vi "CIPT_softwarecontrol auto probe 9 8 23.vi"() -> ()   [LabVIEW 2022 SP3]
uses:
  Git/CIPT/CIPT/Labview Project/CIPT modes.ctl
  <vilib>/Analysis/baseanly.llb/Mean (DBL).vi
  <vilib>/Utility/file.llb/Read Delimited Spreadsheet (DBL).vi
  <vilib>/Utility/file.llb/Read Delimited Spreadsheet (I64).vi
  <vilib>/gmath/NumericalOptimization/Nonlinear Curve Fit LM.vi
  <vilib>/Utility/file.llb/Write Delimited Spreadsheet (string).vi
  <vilib>/Utility/file.llb/Write Delimited Spreadsheet (I64).vi
  <vilib>/Utility/file.llb/Write Delimited Spreadsheet (DBL).vi
  C:/CIPT/Labview Project/Camera Driver/Labview Driver/OtherDrivers/LabVIEW/ueye.NET/uEyeDotNet.dll
  CIPT/Labview Project/Camera Driver/Labview Driver/OtherDrivers/LabVIEW/ueye.NET/uEyeDotNet.dll
  <vilib>/gmath/NI_Gmath.lvlib
  <instrlib>/Keithley DMM6500 DAQ6500 Series/Keithley DMM6500 DAQ6500 Series.lvlib
  <instrlib>/Keithley 24XX/Keithley 24XX.lvlib
  <instrlib>/Keithley 2182/Keithley 2182.lvlib
  <vilib>/Analysis/NI_AALBase.lvlib
panel:
  out "Comms Errors":errorcluster[](array[cluster])
  in  "Save File":bool
  out "error file out":errorcluster
  in  "output file path":path=path "C:/CIPT/Labview Project/csv files/test output.csv"
  in  "stop":bool
  in  "Tab Control":T1(tab)
  in  "Camera ID 3":enum16{"2", "1"}(ring)
  in  "Camera ID 1":enum16{"2", "1"}(ring)
  in  "down a2":bool
  in  "up a2":bool
  in  "down a1":bool
  in  "up a1":bool
  in  "down a3":bool
  in  "up a3":bool
  in  "down all":bool
  in  "up all":bool
  in  "steps /\n continuous \ntoggle":bool
  out "Image first camera":picture
  out "Serial Number 1":string
  in  "Init Camera":bool
  in  "Exit Camera":bool
  in  "Init Camera 2":bool
  in  "Exit Camera 2":bool
  out "Serial Number 2":string
  out "Image second camera":picture
  out "Error Camera 1":errorcluster caption="error"
  out "Error Camera 2":errorcluster caption="error"
  in  "COM 1 (motor)":refnum<visa-resource-name>="COM1"
  out "error":errorcluster
  in  "Turn On Landing Test":bool
  in  "Step size":i32=10
  in  "Probe Landing File":path=path "C:/CIPT/Labview Project/csv files/Probe Landing cipt.csv"
  out "List Of Probe Configs":i64[][](array[numeric])
  out "Resistance For Each Relay Config":sgl[](array[numeric])
  in  "Probe Threshold (ohm)":dbl=100000.0
  out "Touching Probes Configs":i64[][](array[numeric])
  in  "Automatically Move Probe to Surface":bool
  out "Loaded":bool
  out "Loaded":bool
  out "Error Probe Configuration File":errorcluster
  in  "Probe Configuration File":path=path "C:/CIPT/Labview Project/csv files/test probe config.csv"
  in  "Probe Settings File":path=path "C:/CIPT/Labview Project/csv files/deafult_probe_setrings.CSV"
  out "Error Probe Settings File":errorcluster
  out "Probe Spacings":dbl[][](array[numeric])
  in  "Load":bool
  in  "Multiplexer":refnum<visa-resource-name>
  out "all rows":i64[][](array[numeric])
  out "Results Description":string[](array[string])
  out "Results":dbl[][](array[numeric])
  out "Probe Set 2":i32
  in  "Compliance voltage (V)":dbl=42.0
  in  "Measure Instrument":refnum<visa-resource-name>
  in  "Radio Buttons":T2 caption="Select Instrumentation"
  in  "Source Instrument":refnum<visa-resource-name>="Sourcemeter"
  in  "Run":bool
  in  "Current (µA)":dbl=10.0
  out "Measurement Log":string
  out "Probe Set":i32
  in  "Measurement Repeats":i32=10
  in  "Size Of Buffer Used For One Measurement":i32=3
  in  "Top Film R est.":dbl=0.25
  in  "Bottm Film R est.":dbl=0.25
  in  "RA est.":dbl=0.25
  out "Top Film R":dbl
  out "Bottom Film R":dbl
  out "RA":dbl
  out "error out (fitting model)":errorcluster
  in  "Fit Data":bool
  out "Measurements Map Out":map{string, dbl[]}(c390)
  # "Probe Landing cipt_probe check: checks probes individually \nProbe Landing cipt: checks for any connection"
  # "All"
  # "End"
  # "Home"
  # "Delete"
  # "Insert"
  # "Page Down"
  # "Page Up"
  # "F2"
  # "F1"
  # "Steps"
  # "Continuous"
  # "Probe Settings"
  # "Probe Configuration"
  # "I+"
  # "V+"
  # "V-"
  # "I-"
  # "Max Resolution of 2400 is 300 µV in 200 mV range"
  # "/"
  # "Sheet Resistance (RA)"
  # "Estimated Values"
  # "Fitted Values"
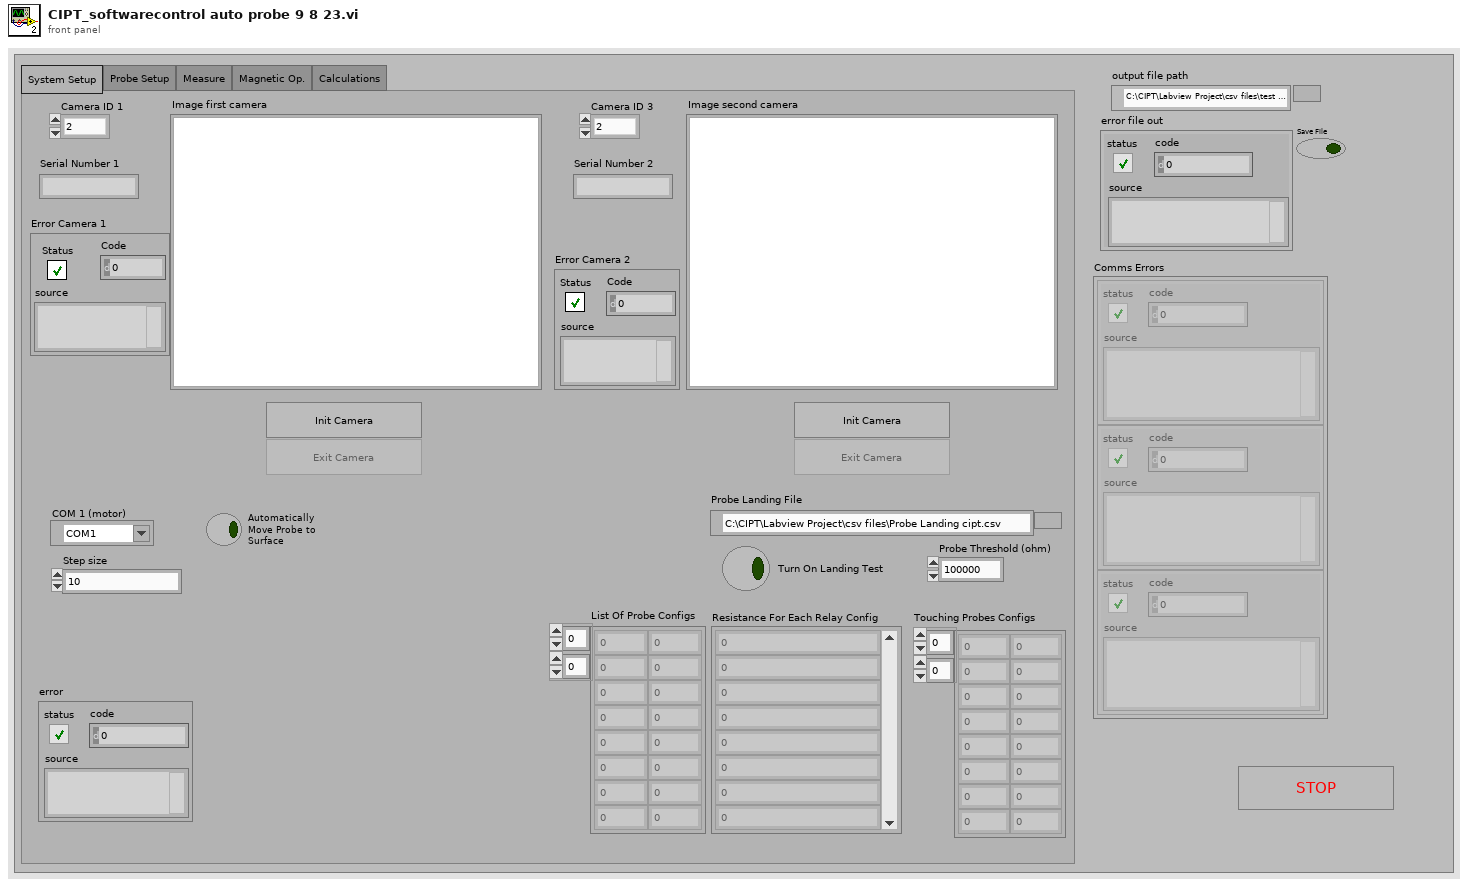
[diagram p1: front panel]
types:
  T1 = enum32{"System Setup", "Probe Setup", "Measure", "Magnetic Op.", "Calculations"}
  T2 = typedef "CIPT modes.ctl" = enum32{"DAQ6510", "2400 Only", "2400 and  2182", "SR830", "SR830 and 6221"}
  T3 = enum32{"System Setup", "Probe Setup", "Measure", "Magnetic Operations", "Calculations + Analyis"}
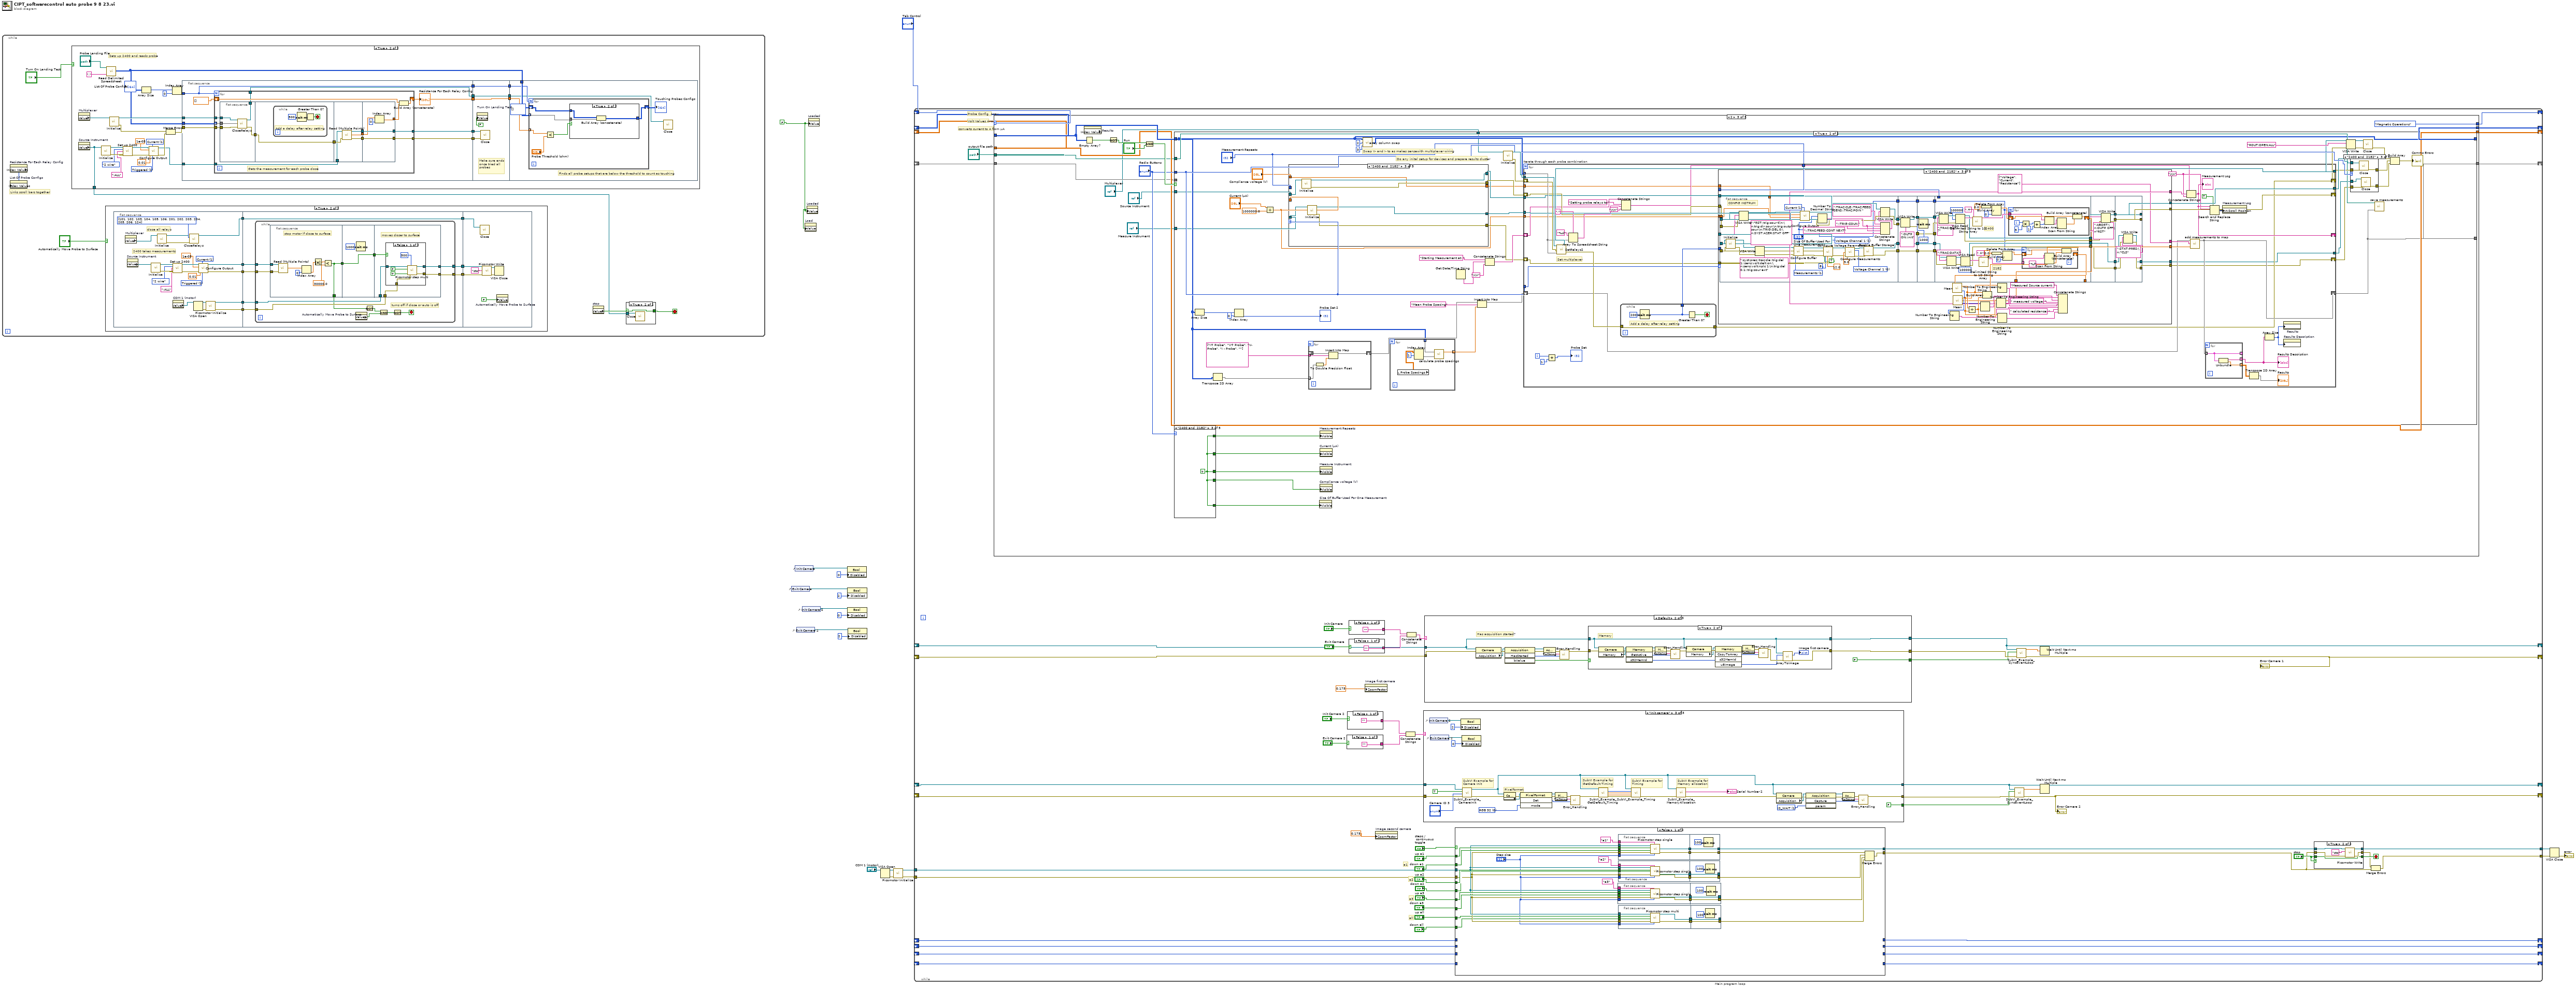
[diagram p0: block diagram]
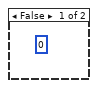
[diagram p5: hidden frame]
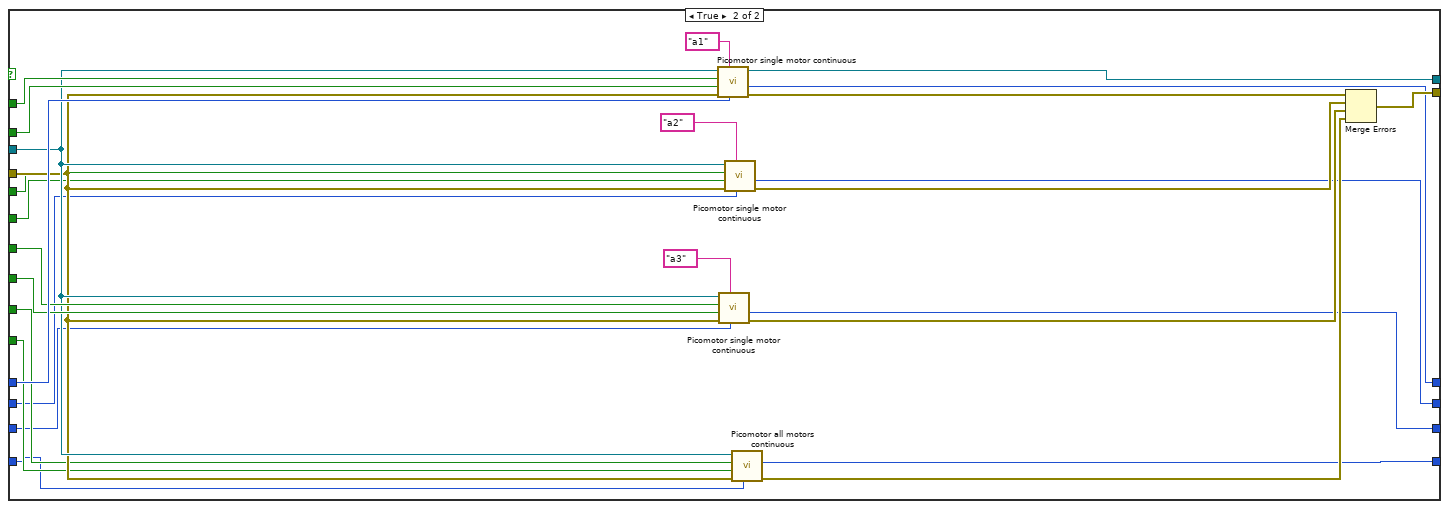
[diagram p7: hidden frame]
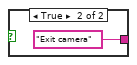
[diagram p9: hidden frame]
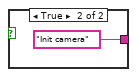
[diagram p10: hidden frame]
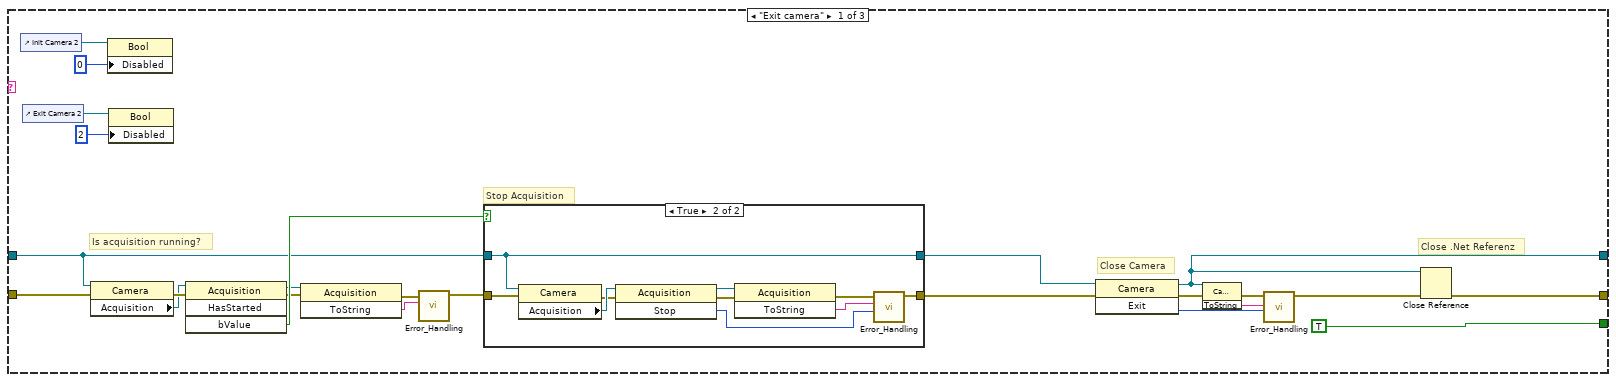
[diagram p11: hidden frame]
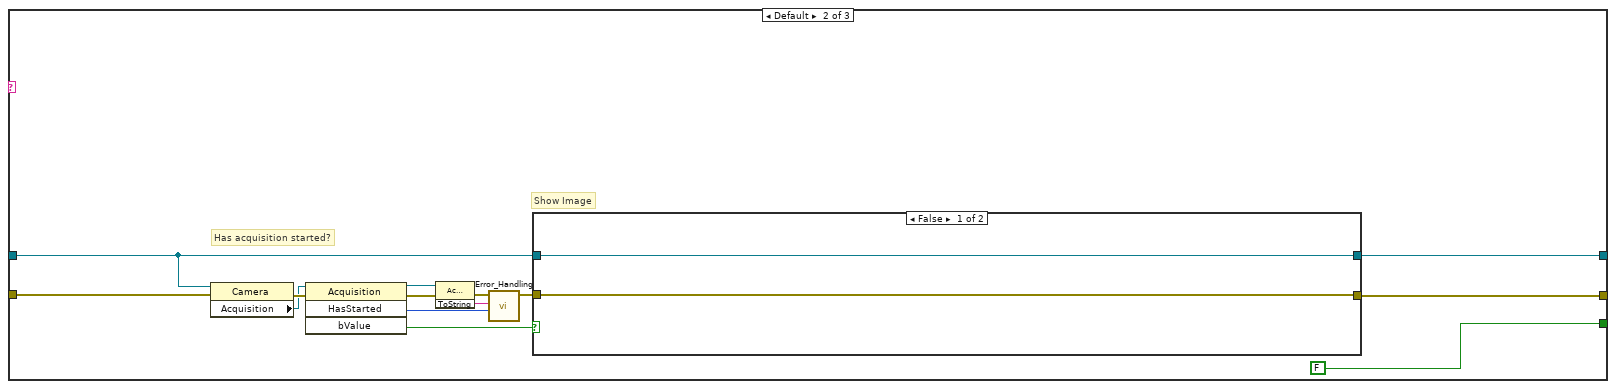
[diagram p13: hidden frame]
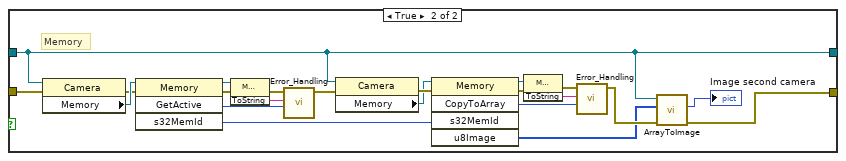
[diagram p14: hidden frame]
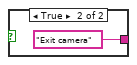
[diagram p15: hidden frame]
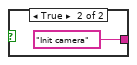
[diagram p16: hidden frame]
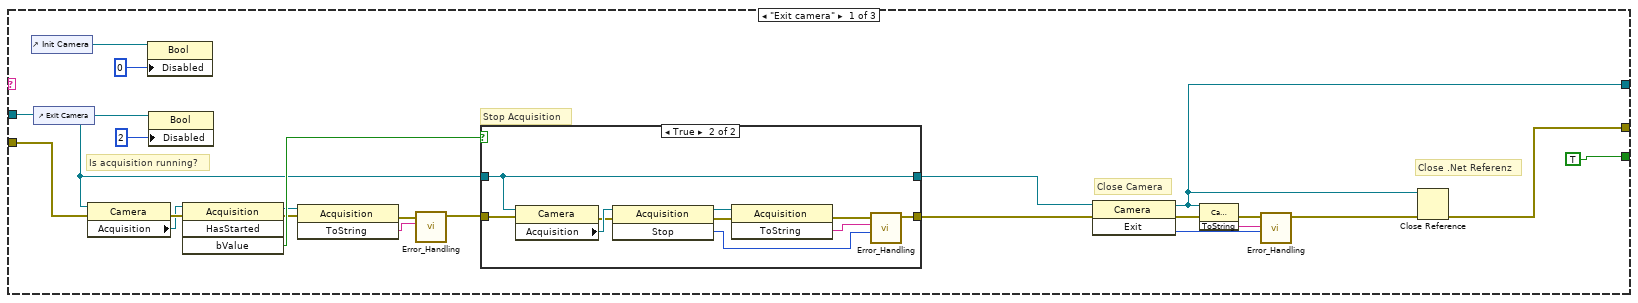
[diagram p17: hidden frame]
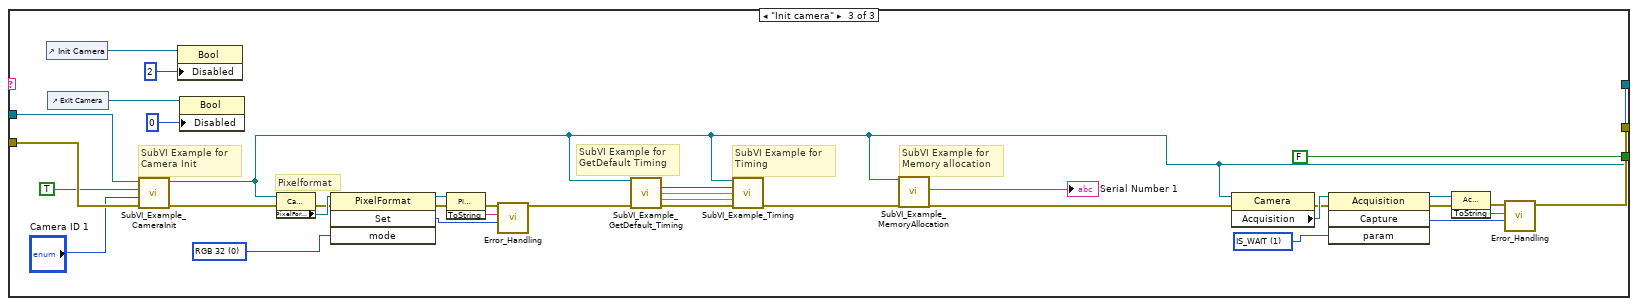
[diagram p20: hidden frame]
diagram:
  w9 = FALSE
  n1 = while {
    stop <- w24 stop-if-true
    # "Links scroll bars together"
    n2 = property on="Resistance For Each Relay Config" class="Arr (strict)"() -> ("Index Values"=w20:u32[])  [unwired: 2 in, 2 out]
    n3 = property on="List Of Probe Configs" class="Arr (strict)"("Index Values"=w20) -> ()  [unwired: 2 in, 2 out]
    n4 = case shown="True" "Turn On Landing Test" {
      tunnel: [_ w117] -> w21
      frame False {
        (unwired) 0
      }
      frame True {
        w134 = u16 1 items=["Immediate", "Triggered"] ("Output Type  (0: Immediate)")
        w133 = u16 1 items=["Voltage", "Current"] ("Source Mode  (0: Voltage)")
        # "Sets up 2400 and reads probe"
        n5 = property on="Multiplexer" class="VISAName"() -> ("Value"=w128:refnum<visa-resource-name>)  [unwired: 2 in, 2 out]
        n6 = property on="Source Instrument" class="VISAName"() -> ("Value"=w117:refnum<visa-resource-name>)  [unwired: 2 in, 2 out]
        n7 = call <instrlib>:"Initialize.vi"("VISA resource name"=w117) -> ("error out"=w136:errorcluster, "VISA resource name out"=w135:refnum<visa-resource-name>)  [unwired: 9 in]
        n8 = call-poly <vilib>:"Read Delimited Spreadsheet.vi"("file path (dialog if empty)"="Probe Landing File", "delimiter (\\t)"="," ("delimiter (\\t)")) -> ("all rows"=w114:i64[][])  [unwired: 8 in, 5 out]
        "List Of Probe Configs" <- w114
        n9 = call <instrlib>:"Initialize.vi"("VISA resource name"=w128) -> ("error out"=w126:errorcluster, "VISA resource name out"=w121:refnum<visa-resource-name>)  [unwired: 9 in]
        n10 = call "Set up 2400.vi"("VISA resource name"=w135, "Sense mode"=enum16{"2 wire", "4 wire"}."2 wire", "Measurement Function"=":ALL", "error in (no error)"=w136) -> ("VISA resource name out"=w137:refnum<visa-resource-name>, "error out"=w138:errorcluster)  [unwired: 10 in]
        n11 = Array Size(array=w114) -> (size(s)=w125:i32[])
        n12 = call <instrlib>:"Configure Output.vi"("Output Type  (0: Immediate)"=w134, "Source Mode  (0: Voltage)"=w133, "error in (no error)"=w138, "Compliance  Level (0.1)"=0.01, "Output Level (0)"=1e-05, "VISA resource name"=w137) -> ("error out"=w127:errorcluster, "VISA resource name out"=w120:refnum<visa-resource-name>)  [unwired: 4 in]
        n13 = Merge Errors(w126, w127) -> (w122:errorcluster)
        n14 = Index Array(array=w125, index=0) -> (element=w123:i32)
        n15 = flat-sequence {
          tunnel: w123 -> [w143]
          tunnel: w122 -> [w150]
          tunnel: w121 -> [w149]
          tunnel: w114 -> [w148]
          tunnel: w120 -> [w147]
          tunnel: [w146] -> w119
          tunnel: [w145] -> w118
          tunnel: [w144] -> w115
          tunnel: [w143] -> w112
          tunnel: [w141] -> w110
          tunnel: w119 -> [w189]
          tunnel: w118 -> [w188]
          tunnel: [w187] -> w116
          tunnel: w115 -> [w187]
          tunnel: [w186] -> w113
          tunnel: w112 -> [w186]
          tunnel: [w185] -> w111
          tunnel: w110 -> [w185]
          tunnel: w116 -> [w196]
          tunnel: w114 -> [w195]
          tunnel: w113 -> [w194]
          tunnel: w111 -> [w191]
          frame #0 {
            n16 = for {
              N: w143 -> [_]
              tunnel: w150 -> [w163]
              tunnel: w149 -> [w162]
              tunnel: w148 -> [w161] mode=indexing
              shift-right: [w156] -> w144
              shift-left: dbl[] [] -> [w155]
              tunnel: w147 -> [w154]
              tunnel: [w153] -> w146
              tunnel: [w152] -> w145
              tunnel: [w151] -> w141
              # "Gets the measurement for each probe close"
              n17 = flat-sequence {
                tunnel: [w170] -> w165
                tunnel: w163 -> [w169]
                tunnel: w162 -> [w168]
                tunnel: w161 -> [w167]
                tunnel: [w166] -> w151
                tunnel: [w171] -> w164
                tunnel: w165 -> [w171]
                tunnel: w164 -> [w179]
                tunnel: [w178] -> w160
                tunnel: [w177] -> w159
                tunnel: [w176] -> w158
                tunnel: w154 -> [w175]
                tunnel: [w183] -> w152
                tunnel: [w184] -> w153
                tunnel: w160 -> [w184]
                tunnel: w159 -> [w183]
                tunnel: w158 -> [w181]
                tunnel: [w180] -> w157
                frame #0 {
                  n18 = call "CloseRelays.vi"("error in (no error)"=w169, "Array"=w167, "VISA Refnum in"=w168) -> ("error out"=w170:errorcluster, "VISA Refnum out"=w166:refnum<visa-resource-name>)  [unwired: 6 in, 1 out]
                }
                frame #1 {
                  n19 = while {
                    stop <- w173 stop-if-true
                    # "Add a delay after relay setting"
                    n20 = Wait (ms)(milliseconds to wait=u32 500) -> (millisecond timer value=w172:u32)
                    n21 = Greater Than 0?(x=w172) -> (x > 0?=w173:bool)
                  }
                }
                frame #2 {
                  n22 = call <instrlib>:"Read (Multiple Points).vi"("VISA resource name"=w175, "error in (no error)"=w179) -> ("VISA resource name out"=w178:refnum<visa-resource-name>, "Resistance"=w176:sgl[], "error out"=w177:errorcluster)  [unwired: 7 in, 4 out]
                }
                frame #3 {
                  n23 = Index Array(array=w181, index=0) -> (element=w180:sgl)
                }
              }
              n24 = Build Array (concatenate)(w155, w157) -> (w156:dbl[])
            }
            "Resistance For Each Relay Config" <- w144
          }
          frame #1 {
            # "Make sure ends once tried all probes"
            n25 = property on="Turn On Landing Test" class="Bool (strict)"("Value"=FALSE) -> ()  [unwired: 2 in, 2 out]
            n26 = call <instrlib>:"Close.vi"("error in (no error)"=w188, "VISA resource name"=w189) -> ()  [unwired: 9 in, 1 out]
          }
          frame #2 {
            # "Finds all probe setups that are below the threshold to count as touching"
            n27 = for {
              N: w194 -> [_]
              tunnel: w196 -> [w201] mode=indexing
              tunnel: w195 -> [w199] mode=indexing
              shift-right: [w198] -> w193
              shift-left: i64[][] [] -> [w197]
              n28 = Less?(x=w201, y="Probe Threshold (ohm)") -> (x < y?=w200:bool)
              n29 = case shown="True" w200 {
                tunnel: w199 -> [_ w206]
                tunnel: [w203 w205] -> w198
                tunnel: w197 -> [w203 w204]
                frame False {
                }
                frame True {
                  n30 = Build Array (concatenate)(w204, w206) -> (w205:i64[][])
                }
              }
            }
            "Touching Probes Configs" <- w193
            n31 = call <instrlib>:"Close.vi"("VISA resource name"=w191) -> ()  [unwired: 10 in, 1 out]
          }
        }
      }
    }
    n32 = case shown="True" "Automatically Move Probe to Surface" {
      frame False {
      }
      frame True {
        n33 = flat-sequence {
          tunnel: [w42] -> w32
          tunnel: [w41] -> w31
          tunnel: [w37] -> w30
          tunnel: [w36] -> w29
          tunnel: [w35] -> w28
          tunnel: w32 -> [w61]
          tunnel: w31 -> [w60]
          tunnel: w30 -> [w59]
          tunnel: w29 -> [w58]
          tunnel: w28 -> [w62]
          tunnel: [w62] -> w27
          tunnel: [w57] -> w26
          tunnel: [w56] -> w25
          tunnel: w27 -> [w101]
          tunnel: w26 -> [w102]
          tunnel: w25 -> [w104]
          frame #0 {
            w51 = u16 1 items=["Immediate", "Triggered"] ("Output Type  (0: Immediate)")
            w33 = u16 1 items=["Voltage", "Current"] ("Source Mode  (0: Voltage)")
            # "2400 takes measurements"
            # "close all relays"
            n34 = property on="Multiplexer" class="VISAName"() -> ("Value"=w46:refnum<visa-resource-name>)  [unwired: 2 in, 2 out]
            n35 = property on="Source Instrument" class="VISAName"() -> ("Value"=w47:refnum<visa-resource-name>)  [unwired: 2 in, 2 out]
            n36 = call <instrlib>:"Initialize.vi"("VISA resource name"=w47) -> ("error out"=w53:errorcluster, "VISA resource name out"=w52:refnum<visa-resource-name>)  [unwired: 9 in]
            n37 = call <instrlib>:"Initialize.vi"("VISA resource name"=w46) -> ("error out"=w43:errorcluster, "VISA resource name out"=w44:refnum<visa-resource-name>)  [unwired: 9 in]
            n38 = call "Set up 2400.vi"("VISA resource name"=w52, "Sense mode"=enum16{"2 wire", "4 wire"}."2 wire", "Measurement Function"=":ALL", "error in (no error)"=w53) -> ("VISA resource name out"=w54:refnum<visa-resource-name>, "error out"=w55:errorcluster)  [unwired: 10 in]
            n39 = property on="COM 1 (motor)" class="VISAName"() -> ("Value"=w40:refnum<visa-resource-name>)  [unwired: 2 in, 2 out]
            n40 = call "CloseRelays.vi"("error in (no error)"=w43, "Array"=i32[] [101, 102, 103, 104, 105, 106, 201, 202, 203, 204, 205, 206, 124], "VISA Refnum in"=w44) -> ("VISA Refnum out"=w35:refnum<visa-resource-name>)  [unwired: 6 in, 2 out]
            n41 = VISA Open(VISA resource name=w40) -> (VISA resource name=w38:refnum<visa-resource-name>, error out=w39:errorcluster)  [unwired: 4 in]
            n42 = call <instrlib>:"Configure Output.vi"("Output Type  (0: Immediate)"=w51, "Source Mode  (0: Voltage)"=w33, "error in (no error)"=w55, "Compliance  Level (0.1)"=0.01, "Output Level (0)"=1e-05, "VISA resource name"=w54) -> ("error out"=w41:errorcluster, "VISA resource name out"=w42:refnum<visa-resource-name>)  [unwired: 4 in]
            n43 = call "Picomotor Initialize.vi"("error in (no error)"=w39, "VISA Refnum in"=w38) -> ("error out"=w36:errorcluster, "VISA Refnum out"=w37:refnum<visa-resource-name>)  [unwired: 8 in]
          }
          frame #1 {
            n44 = while {
              tunnel: w61 -> [w75]
              tunnel: w60 -> [w74]
              tunnel: w59 -> [w73]
              tunnel: w58 -> [w72]
              tunnel: [w71] -> w57
              tunnel: [w70] -> w56
              stop <- w63 stop-if-true
              # "turns off if close or auto is off"
              n45 = flat-sequence {
                tunnel: w75 -> [w81]
                tunnel: w74 -> [w80]
                tunnel: [w78] -> w67
                tunnel: [w78] -> w68
                tunnel: [w84] -> w69
                tunnel: w68 -> [w84]
                tunnel: w73 -> [w89]
                tunnel: w72 -> [w90]
                tunnel: [w87] -> w71
                tunnel: [w88] -> w70
                tunnel: w69 -> [w86]
                frame #0 {
                  # "stop motor if close to surface"
                  n46 = call <instrlib>:"Read (Multiple Points).vi"("VISA resource name"=w81, "error in (no error)"=w80) -> ("Resistance"=w82:sgl[])  [unwired: 7 in, 6 out]
                  n47 = Index Array(array=w82, index=0) -> (element=w77:sgl)
                  n48 = Absolute Value(x=w77) -> (abs(x)=w76:sgl)
                  n49 = Less?(x=w76, y=sgl 30000.0 ("x")) -> (x < y?=w78:bool)
                }
                frame #1 {
                  n50 = Wait (ms)(milliseconds to wait=u32 1000) -> ()  [unwired: 1 out]
                }
                frame #2 {
                  # "moves closer to surface"
                  n51 = case shown="False" w86 {
                    tunnel: w90 -> [w96 w98]
                    tunnel: w89 -> [w93 w99]
                    tunnel: [w92 w98] -> w88
                    tunnel: [w91 w99] -> w87
                    frame False {
                      n52 = call "Picomotor step multi.vi"("Step size"=500, "error in (no error)"=w96, "down a1"=TRUE, "up a1"=FALSE, "VISA Refnum in"=w93) -> ("error out"=w92:errorcluster, "VISA Refnum out"=w91:refnum<visa-resource-name>)  [unwired: 5 in]
                    }
                    frame True {
                    }
                  }
                }
              }
              n53 = property on="Automatically Move Probe to Surface" class="Bool (strict)"() -> ("Value"=w66:bool)  [unwired: 2 in, 2 out]
              n54 = Not(x=w67) -> (.not. x?=w65:bool)
              n55 = And(x=w65, y=w66) -> (x .and. y?=w64:bool)
              n56 = Not(x=w64) -> (.not. x?=w63:bool)
            }
          }
          frame #2 {
            n57 = call <instrlib>:"Close.vi"("VISA resource name"=w101) -> ()  [unwired: 10 in, 1 out]
            n58 = call "Picomotor Write.vi"("error in (no error)"=w104, "String 3"="sto", "VISA Refnum in"=w102) -> ("error out"=w106:errorcluster, "VISA Refnum out"=w105:refnum<visa-resource-name>)  [unwired: 6 in, 1 out]
            n59 = VISA Close(VISA resource name=w105, error in (no error)=w106) -> ()  [unwired: 1 out]
            n60 = property on="Automatically Move Probe to Surface" class="Bool (strict)"("Value"=FALSE) -> ()  [unwired: 2 in, 2 out]
          }
        }
      }
    }
    n61 = property on="stop" class="Bool (strict)"() -> ("Value"=w22:bool)  [unwired: 2 in, 2 out]
    n62 = case shown="True" w22 {
      selector: w22 -> [w107 w109]
      tunnel: [w107 w109] -> w24
      tunnel: w21 -> [_ w108]
      frame False {
      }
      frame True {
        n63 = call <instrlib>:"Close.vi"("VISA resource name"=w108) -> ()  [unwired: 10 in, 1 out]
      }
    }
  }
  n64 = control-ref of="Exit Camera"() -> (w12:refnum<vi>)
  n65 = control-ref of="Init Camera"() -> (w13:refnum<vi>)
  n66 = control-ref of="Exit Camera 2"() -> (w17:refnum<vi>)
  n67 = control-ref of="Init Camera 2"() -> (w16:refnum<vi>)
  n68 = property on="Load" class="Bool (strict)"("Value"=w9) -> ()  [unwired: 2 in, 2 out]
  n69 = property on="Loaded" class="Bool (strict)"("Value"=w9) -> ()  [unwired: 2 in, 2 out]
  n70 = property on="Loaded" class="Bool (strict)"("Value"=w9) -> ()  [unwired: 2 in, 2 out]
  n71 = property class="Bool"(reference=w13, "Disabled"=u8 0 ("Deaktiviert")) -> ()  [unwired: 1 in, 2 out]
  n72 = property class="Bool"(reference=w12, "Disabled"=u8 2 ("Deaktiviert")) -> ()  [unwired: 1 in, 2 out]
  n73 = property class="Bool"(reference=w16, "Disabled"=u8 0 ("Deaktiviert")) -> ()  [unwired: 1 in, 2 out]
  n74 = property class="Bool"(reference=w17, "Disabled"=u8 2 ("Deaktiviert")) -> ()  [unwired: 1 in, 2 out]
  n75 = VISA Open(VISA resource name="COM 1 (motor)") -> (VISA resource name=w7:refnum<visa-resource-name>, error out=w6:errorcluster)  [unwired: 4 in]
  n76 = call "Picomotor Initialize.vi"("error in (no error)"=w6, "VISA Refnum in"=w7) -> ("error out"=w4:errorcluster, "VISA Refnum out"=w5:refnum<visa-resource-name>)  [unwired: 8 in]
  n77 = while "Main program loop" {
    shift-right: [w265] -> _
    shift-left: _ -> [w266]
    shift-right: [w264] -> _
    shift-left: "Tab Control" -> [w267]
    shift-right: [w263] -> _
    shift-left: _ -> [w262]
    shift-right: [w260] -> _
    shift-left: _ -> [w259]
    shift-right: [w248] -> _
    shift-left: _ -> [w246]
    shift-right: [w249] -> _
    shift-left: _ -> [w247]
    shift-right: [w236] -> _
    shift-left: _ -> [w234]
    shift-right: [w235] -> _
    shift-left: _ -> [w233]
    tunnel: w5 -> [w220]
    tunnel: w4 -> [w219]
    tunnel: [w232] -> w2
    shift-right: [w217] -> _
    shift-left: _ -> [w213]
    shift-right: [w216] -> _
    shift-left: _ -> [w212]
    shift-right: [w215] -> _
    shift-left: _ -> [w211]
    shift-right: [w214] -> _
    shift-left: _ -> [w210]
    tunnel: [w207] -> w1
    stop <- w231 stop-if-true
    # "a2"
    # "a3"
    # "all"
    # "a1"
    # "converts current to A from µA"
    # "Volt Values Array"
    # "Probe Config. Array"
    n78 = case shown="2" w267 {
      tunnel: w266 -> [w606 w613 w643 w1002 w1009]
      tunnel: [w606 w617 w642 w1002 w1009] -> w265
      tunnel: [T3."Probe Setup" ("Tab Control") T3."Measure" ("Tab Control") T3."Magnetic Operations" ("Tab Control") T3."Calculations + Analyis" ("Tab Control") T3."System Setup" ("Tab Control")] -> w264
      tunnel: [w604 w612 w637 w1001 w1008] -> w263
      tunnel: w262 -> [w604 w611 w637 w1001 w1008]
      tunnel: "output file path" -> [_ _ w634 _ w1007]
      tunnel: [w603 w608 w633 w1000 w1006] -> w260
      tunnel: w259 -> [w603 w608 w632 w1000 w1006]
      frame 0, Default {
        # "System Setup"
      }
      frame 1 {
        # "Probe Setup"
        n79 = Empty Array?(array=w613) -> (empty?=w607:bool)
        n80 = Empty Array?(array=w611) -> (empty?=w610:bool)
        n81 = Not(x=w607) -> (.not. x?=→"Loaded":bool)
        n82 = Not(x=w610) -> (.not. x?=→"Loaded":bool)
        n83 = case shown="True" "Load" {
          tunnel: [w619 w620] -> w617
          tunnel: w613 -> [w619 _]
          tunnel: [w618 w621] -> w612
          tunnel: w611 -> [w618 _]
          frame False {
          }
          frame True {
            # "Probe config. file and data aquisition"
            # "Probe settings file and data aquisition"
            n84 = call-poly <vilib>:"Read Delimited Spreadsheet.vi"("file path (dialog if empty)"="Probe Configuration File", "delimiter (\\t)"="," ("delimiter (\\t)")) -> ("all rows"=w620:i64[][], "error out"=→"Error Probe Configuration File":errorcluster)  [unwired: 8 in, 4 out]
            "all rows" <- w620
            n85 = call-poly <vilib>:"Read Delimited Spreadsheet.vi"("file path (dialog if empty)"="Probe Settings File", "delimiter (\\t)"="," ("delimiter (\\t)")) -> ("all rows"=w621:dbl[][], "error out"=→"Error Probe Settings File":errorcluster)  [unwired: 8 in, 4 out]
            "Probe Spacings" <- w621
          }
        }
        n86 = property on="Load" class="Bool (strict)"("Value"=w607) -> ()  [unwired: 2 in, 2 out]
      }
      frame 2 {
        n87 = property on="Results" class="Arr (strict)" props=["Index Values"]() -> ()  [unwired: 2 in, 3 out]
        n88 = Empty Array?(array=w643) -> (empty?=w645:bool)
        n89 = Not(x=w645) -> (.not. x?=w644:bool)
        n90 = Compound Arithmetic op=AND(w644, "Run") -> (w647:bool)
        n91 = case shown="True" w647 {
          tunnel: w643 -> [w658 w677]
          tunnel: [w658 w677] -> w642
          tunnel: "Radio Buttons" -> [_ w703]
          tunnel: w634 -> [_ w691]
          tunnel: [w657 w673] -> w633
          tunnel: w632 -> [w657 _]
          tunnel: "Measure Instrument" -> [_ w665]
          tunnel: "Source Instrument" -> [_ w664]
          tunnel: "Multiplexer" -> [_ w663]
          frame False {
          }
          frame True {
            # "Swap V- and I- to as makes sensewith multiplexer wiring"
            # "Do any inital setup for devices and prepare results cluster"
            n92 = Array Size(array=w677) -> (size(s)=w697:i32[])
            n93 = Transpose 2D Array(2D array=w677) -> (transposed array=w676:i64[][])
            n94 = Index Array "Index Array"(array=w697, index=0) -> (element=→"Probe Set 2":i32)
            n95 = Divide(x="Current (µA)", y=1000000.0) -> (x/y=w659:dbl)
            n96 = case shown="\"2400 and  2182\"" w703 {
              tunnel: w664 -> [_ w741 w747 _ _]
              tunnel: [_ w729 w746 _ _] -> w704
              tunnel: w665 -> [_ _ w748 _ _]
              tunnel: [_ w729 w744 _ _] -> w667
              tunnel: [_ w735 w743 _ _] -> w698
              tunnel: w659 -> [_ w732 _ _ _]
              tunnel: "Compliance voltage (V)" -> [_ w730 w742 _ _]
              tunnel: "Measurement Repeats" -> [_ _ _ _ _]
              tunnel: [_ _ w745 _ _] -> w662
              tunnel: [_ _ w742 _ _] -> w660
              frame "DAQ6510", Default {
              }
              frame "2400 Only" {
                w733 = u16 1 items=["Immediate", "Triggered"] ("Output Type  (0: Immediate)")
                w734 = u16 1 items=["Voltage", "Current"] ("Source Mode  (0: Voltage)")
                n97 = call <instrlib>:"Initialize.vi"("VISA resource name"=w741) -> ("error out"=w739:errorcluster, "VISA resource name out"=w740:refnum<visa-resource-name>)  [unwired: 9 in]
                n98 = call "Set up 2400.vi"("VISA resource name"=w740, "Sense mode"=enum16{"2 wire", "4 wire"}."4 wire", "Measurement Function"=":ALL", "error in (no error)"=w739) -> ("VISA resource name out"=w737:refnum<visa-resource-name>, "error out"=w736:errorcluster)  [unwired: 10 in]
                n99 = call <instrlib>:"Configure Output.vi"("Output Type  (0: Immediate)"=w733, "Source Mode  (0: Voltage)"=w734, "error in (no error)"=w736, "Compliance  Level (0.1)"=w730, "Output Level (0)"=w732, "VISA resource name"=w737) -> ("error out"=w735:errorcluster, "VISA resource name out"=w729:refnum<visa-resource-name>)  [unwired: 4 in]
              }
              frame "2400 and  2182" {
                n100 = call <instrlib>:"Initialize.vi"("VISA resource name"=w747) -> ("error out"=w743:errorcluster, "VISA resource name out"=w744:refnum<visa-resource-name>)  [unwired: 9 in]
                n101 = call <instrlib>:"Initialize.vi"("VISA resource name"=w748) -> ("error out"=w745:errorcluster, "VISA resource name out"=w746:refnum<visa-resource-name>)  [unwired: 9 in]
              }
              frame "SR830" {
              }
              frame "SR830 and 6221" {
              }
            }
            n102 = for {
              tunnel: w676 -> [w715] mode=indexing
              tunnel: string[] ["I+ Probe", "V+ Probe", "V- Probe", "I - Probe", ""] -> [w716] mode=indexing
              shift-right: [w713] -> w681
              shift-left: _ -> [w712]
              n103 = To Double Precision Float(number=w715) -> (double precision float=w714:dbl[])
              n104 = Insert Into Map(map in=w712, key=w716, value=w714) -> (map out=w713:map{string, dbl[]})  [unwired: 2 out]
            }
            n105 = call "array column swap.vi"("Collumn 2 index"=3, "Collumn 1 index"=2, "Input array"=w677) -> ("output array"=w694:i32[][])
            n106 = for {
              tunnel: w677 -> [w708] mode=indexing
              tunnel: [w707] -> w680 mode=indexing
              n107 = local read "Probe Spacings"() -> (w711:dbl[][])
              n108 = Index Array(array=w711, index (row)=1) -> (element=w709:dbl[])  [unwired: 1 in]
              n109 = call "calculate probe spacings.vi"("Probe Spacings"=w709, "Probe list"=w708) -> ("Mean Spacing"=w707:dbl)  [unwired: 1 out]
            }
            n110 = Get Date/Time String() -> (time string=w700:string)  [unwired: 3 in, 1 out]
            n111 = Insert Into Map(map in=w681, key="Mean Probe Spacing", value=w680) -> (map out=w678:map{string, dbl[]})  [unwired: 2 out]
            n112 = Concatenate Strings("Starting Measurement at: ", w700, "\r\n") -> (w689:string)
            n113 = call <instrlib>:"Initialize.vi"("VISA resource name"=w663) -> ("error out"=w705:errorcluster, "VISA resource name out"=w706:refnum<visa-resource-name>)  [unwired: 9 in]
            n114 = for "Iterate through each probe combination" {
              tunnel: w706 -> [w790]
              tunnel: [w789] -> w687
              tunnel: w694 -> [w783] mode=indexing
              tunnel: w703 -> [w788]
              tunnel: w704 -> [w786]
              shift-right: [w772] -> _
              shift-left: w689 -> [w773]
              shift-right: [w784] -> w701
              shift-left: w698 -> [w777]
              shift-right: [w763] -> w673
              shift-left: w678 -> [w765]
              shift-right: [w757] -> w674
              shift-left: w662 -> [w758]
              tunnel: w667 -> [w776]
              tunnel: [w785] -> w702
              shift-right: [w760] -> w669
              shift-left: w705 -> [w787]
              tunnel: [w756] -> w675
              tunnel: "Measurement Repeats" -> [w755]
              tunnel: w660 -> [w751]
              tunnel: w659 -> [w750]
              i -> [w754]
              w770 = "\r\n"
              # "Set multiplexer"
              n115 = Add(x=w754, y=1) -> (x+y=→"Probe Set":i32)
              n116 = call "SetRelays2.vi"("all rows"=w783, "error in (no error)"=w787, "VISA Refnum in"=w790) -> ("error out"=w778:errorcluster, "VISA resource name out"=w789:refnum<visa-resource-name>)  [unwired: 1 in]
              n117 = Array To Spreadsheet String(delimiter (Tab)=",", array=w783, 3:"%d" ("format string")) -> (spreadsheet string=w779:string)
              n118 = while {
                tunnel: [w797] -> w760
                tunnel: w778 -> [w797]
                tunnel: [w794] -> w759
                stop <- w795 stop-if-true
                # "Add a delay after relay setting"
                n119 = Wait (ms)(milliseconds to wait=u32 200) -> (millisecond timer value=w794:u32)
                n120 = Greater Than 0?(x=w794) -> (x > 0?=w795:bool)
              }
              n121 = Concatenate Strings(w773, "Setting probe relays to:", w779, "\r\n") -> (w768:string)
              n122 = case shown="\"2400 and  2182\"" w788 {
                tunnel: w786 -> [w799 w803 w868 w992 w996]
                tunnel: w776 -> [w798 w824 w876 w993 w997]
                tunnel: w777 -> [w800 w823 w875 w994 w998]
                tunnel: [w798 w821 w836 w993 w997] -> w785
                tunnel: [w800 w820 w844 w994 w998] -> w784
                tunnel: [_ w813 w869 _ _] -> w774
                tunnel: w755 -> [_ w812 w874 _ _]
                tunnel: [_ w806 w873 _ _] -> w766
                tunnel: [_ string[] ["Voltage", "Current", "Resistance"] string[] ["Voltage", "Current", "Resistance"] _ _] -> w767
                tunnel: w759 -> [_ _ _ _ _]
                tunnel: w758 -> [w801 w804 w867 w995 w999]
                tunnel: [w801 w804 w840 w995 w999] -> w757
                tunnel: [w799 w803 w837 w992 w996] -> w756
                tunnel: w751 -> [_ _ w829 _ _]
                tunnel: w750 -> [_ _ w828 _ _]
                frame "DAQ6510", Default {
                }
                frame "2400 Only" {
                  w822 = u16 0 items=["Fixed", "Sweep", "List"] ("Output Mode (0: Fixed)")
                  n123 = call <instrlib>:"Read (Multiple Points).vi"("VISA resource name"=w824, "Sample Count (1)"=w812, "error in (no error)"=w823, "Output Mode (0: Fixed)"=w822) -> ("Voltage"=w802:sgl[], "VISA resource name out"=w821:refnum<visa-resource-name>, "Current"=w811:sgl[], "Resistance"=w810:sgl[], "error out"=w820:errorcluster)  [unwired: 5 in, 2 out]
                  n124 = call-poly <vilib>:"Mean.vi"("X"=w802) -> ("mean"=w809:dbl)  [unwired: 1 out]
                  n125 = call-poly <vilib>:"Mean.vi"("X"=w811) -> ("mean"=w808:dbl)  [unwired: 1 out]
                  n126 = call-poly <vilib>:"Mean.vi"("X"=w810) -> ("mean"=w807:dbl)  [unwired: 1 out]
                  n127 = Build Array(w809, w808, w807) -> (w806:dbl[])
                  n128 = Number To Engineering String(4:w809) -> (0:w814:string)  [unwired: 3 in]
                  n129 = Number To Engineering String(4:w808) -> (0:w818:string)  [unwired: 3 in]
                  n130 = Number To Engineering String(4:w807) -> (0:w815:string)  [unwired: 3 in]
                  n131 = Concatenate Strings("Measured I = ", w818, " V = " ("string"), w814, "R = " ("string"), w815) -> (w813:string)
                }
                frame "2400 and  2182" {
                  n132 = flat-sequence {
                    tunnel: w867 -> [w883]
                    tunnel: w868 -> [w884]
                    tunnel: w875 -> [w885]
                    tunnel: w876 -> [w886]
                    tunnel: [w890] -> w839
                    tunnel: [w889] -> w838
                    tunnel: [w888] -> w831
                    tunnel: [w887] -> w830
                    tunnel: w829 -> [w881]
                    tunnel: w828 -> [w880]
                    tunnel: ["Size Of Buffer Used For One Measurement"] -> w825
                    tunnel: [w923] -> w856
                    tunnel: [w922] -> w854
                    tunnel: [w920] -> w851
                    tunnel: [w919] -> w849
                    tunnel: w839 -> [w923]
                    tunnel: w838 -> [w922]
                    tunnel: w831 -> [w921]
                    tunnel: w830 -> [_]
                    tunnel: [w917] -> w826
                    tunnel: w825 -> [w917]
                    tunnel: w856 -> [w929]
                    tunnel: [w929] -> w855
                    tunnel: w854 -> [w928]
                    tunnel: [w928] -> w853
                    tunnel: [w926] -> w852
                    tunnel: w851 -> [w926]
                    tunnel: [w925] -> w850
                    tunnel: w849 -> [w925]
                    tunnel: [w924] -> w827
                    tunnel: w826 -> [w924]
                    tunnel: w874 -> [_]
                    tunnel: w855 -> [w939]
                    tunnel: w853 -> [w938]
                    tunnel: w852 -> [w941]
                    tunnel: w850 -> [w940]
                    tunnel: [w937] -> w848
                    tunnel: [w936] -> w847
                    tunnel: [w934] -> w846
                    tunnel: [w933] -> w845
                    tunnel: [w932] -> w842
                    tunnel: [w931] -> w841
                    tunnel: w827 -> [w930]
                    tunnel: w846 -> [w984]
                    tunnel: w845 -> [w983]
                    tunnel: w842 -> [w979]
                    tunnel: w841 -> [w980]
                    tunnel: [w981] -> w835
                    tunnel: [w980] -> w834
                    tunnel: [w979] -> w833
                    tunnel: [w978] -> w832
                    tunnel: [w990] -> w836
                    tunnel: [w985] -> w837
                    tunnel: [w986] -> w840
                    tunnel: [w991] -> w844
                    tunnel: w835 -> [w991]
                    tunnel: w834 -> [w987]
                    tunnel: w833 -> [w988]
                    tunnel: w832 -> [w990]
                    frame #0 {
                      w894 = 0 items=["Voltage Channel 1", "Voltage Channel 2", "Temperature Channel 1", "Temperature Channel 2"] ("Measurement (0: Voltage Channel 1)")
                      w882 = u16 1 items=["Voltage", "Current"] ("Source Mode  (0: Voltage)")
                      w907 = 1 items=["Voltage Channel 1"=1, "Voltage Channel 2"=2] ("Measurement (1: Voltage Channel 1)")
                      w908 = 1 items=["None", "Measurements", "Math Calculation"] ("Buffer Source (0: None)")
                      # "CONFIG INSTRUM"
                      n133 = call <instrlib>:"Initialize.vi"("error in (no error)"=w883, "VISA resource name"=w884) -> ("error out"=w892:errorcluster, "VISA resource name out"=w893:refnum<visa-resource-name>)  [unwired: 8 in]
                      n134 = VISA Write(VISA resource name=w886, write buffer=":*RST;:trig:sour tlin;\n:trig:dir sour;\n:trig:outp sour;\n:TRIG:DEL 0;\n:SYST:AZER:STAT OFF", error in (no error)=w885) -> (VISA resource name out=w903:refnum<visa-resource-name>, error out=w898:errorcluster)  [unwired: 1 out]
                      n135 = VISA Write(VISA resource name=w893, write buffer=":syst:pres;:trac:cle;:trig:del 1;:sens:volt:delt on;\n:sens:volt:nplc 1;\n:trig:del 0.1;:trig:sour ext", error in (no error)=w892) -> (VISA resource name out=w905:refnum<visa-resource-name>, error out=w904:errorcluster)  [unwired: 1 out]
                      n136 = call <instrlib>:"Configure Buffer.vi"("error in (no error)"=w904, "Buffer Source (0: None)"=w908, "Buffer Size (2)"="Size Of Buffer Used For One Measurement", "VISA resource name"=w905) -> ("error out"=w909:errorcluster, "VISA resource name out"=w912:refnum<visa-resource-name>)  [unwired: 6 in]
                      n137 = call <instrlib>:"Configure Output.vi"("Source Mode  (0: Voltage)"=w882, "error in (no error)"=w898, "Compliance  Level (0.1)"=w881, "Output Level (0)"=w880, "VISA resource name"=w903) -> ("error out"=w897:errorcluster, "VISA resource name out"=w879:refnum<visa-resource-name>)  [unwired: 5 in]
                      n138 = Number To Decimal String(number="Size Of Buffer Used For One Measurement") -> (decimal integer string=w899:string)  [unwired: 1 in]
                      n139 = call <instrlib>:"Configure Voltage Parameters.vi"("VISA resource name"=w912, "Measurement (1: Voltage Channel 1)"=w907, "Voltage Resolution (8)"=8, "Range Value (12)"=12.0, "Autorange (T: Enable)"=TRUE, "error in (no error)"=w909) -> ("VISA resource name out"=w911:refnum<visa-resource-name>, "error out"=w910:errorcluster)  [unwired: 8 in]
                      n140 = call <instrlib>:"Configure Measurements.vi"("VISA resource name"=w911, "Measurement (0: Voltage Channel 1)"=w894, "Integration Rate (5)"=5.0, "error in (no error)"=w910) -> ("VISA resource name out"=w896:refnum<visa-resource-name>, "error out"=w895:errorcluster)  [unwired: 10 in]
                      n141 = call <instrlib>:"Enable Buffer Storage.vi"("error in (no error)"=w895, "VISA resource name"=w896) -> ("error out"=w889:errorcluster, "VISA resource name out"=w890:refnum<visa-resource-name>)  [unwired: 8 in]
                      n142 = Concatenate Strings(":TRAC:CLE;:TRAC:FEED SENS;:TRAC:POIN " ("write buffer"), w899, ";:TRIG:COUN " ("write buffer"), w899, ";:TRAC:FEED:CONT NEXT" ("write buffer")) -> (w878:string)
                      n143 = VISA Write(VISA resource name=w879, write buffer=w878, error in (no error)=w897) -> (VISA resource name out=w888:refnum<visa-resource-name>, error out=w887:errorcluster)  [unwired: 1 out]
                    }
                    frame #1 {
                      n144 = VISA Write(VISA resource name=w921, write buffer=":OUTP ON;:init") -> (VISA resource name out=w920:refnum<visa-resource-name>, error out=w919:errorcluster)  [unwired: 1 in, 1 out]
                    }
                    frame #2 {
                      n145 = Wait (ms)(milliseconds to wait=u32 1000) -> ()  [unwired: 1 out]
                    }
                    frame #3 {
                      # "2182"
                      # "2400"
                      n146 = VISA Write(VISA resource name=w941, write buffer=":TRAC:DATA?", error in (no error)=w940) -> (VISA resource name out=w951:refnum<visa-resource-name>, error out=w950:errorcluster)  [unwired: 1 out]
                      n147 = VISA Write(VISA resource name=w939, write buffer=":TRAC:DATA?", error in (no error)=w938) -> (VISA resource name out=w960:refnum<visa-resource-name>, error out=w959:errorcluster)  [unwired: 1 out]
                      n148 = VISA Read(VISA resource name=w951, byte count=u32 100000, error in (no error)=w950) -> (VISA resource name out=w934:refnum<visa-resource-name>, read buffer=w947:string, error out=w933:errorcluster)  [unwired: 1 out]
                      n149 = VISA Read(VISA resource name=w960, byte count=u32 100000, error in (no error)=w959) -> (VISA resource name out=w932:refnum<visa-resource-name>, read buffer=w957:string, error out=w931:errorcluster)  [unwired: 1 out]
                      n150 = call <vilib>:"Delimited String to 1D String Array.vi"("delimiter"=",+" ("delimiter (Tab)"), "delimited string"=w947) -> ("string array"=w943:string[])  [unwired: 9 in]
                      n151 = call <vilib>:"Delimited String to 1D String Array.vi"("delimiter"=",+" ("delimiter (Tab)"), "delimited string"=w957) -> ("string array"=w952:string[])  [unwired: 9 in]
                      n152 = Build Array(0.0 ("array")) -> (w945:dbl[])
                      n153 = Build Array(0.0 ("array")) -> (w955:dbl[])
                      n154 = Delete From Array(array=w945, index=0) -> (array with subset deleted=w935:dbl[])  [unwired: 1 in, 1 out]
                      n155 = Delete From Array(array=w955, index=0) -> (array with subset deleted=w953:dbl[])  [unwired: 1 in, 1 out]
                      n156 = for {
                        N: w930 -> [_]
                        shift-right: [w966] -> w936
                        shift-left: w935 -> [w965]
                        tunnel: w943 -> [w964]
                        i -> [w972]
                        n157 = Multiply(x=w972, y=5) -> (x*y=w971:i32)
                        n158 = Add(x=w971, y=1) -> (x+y=w968:i32)
                        n159 = Index Array(array=w964, index=w968) -> (element=w963:string)
                        n160 = Scan From String(input string=w963) -> (output 1=w967:dbl)  [unwired: 4 in, 3 out]
                        n161 = Build Array (concatenate)(w965, w967) -> (w966:dbl[])
                      }
                      n162 = for {
                        N: w930 -> [_]
                        shift-right: [w975] -> w937
                        shift-left: w953 -> [w974]
                        tunnel: w952 -> [w973] mode=indexing
                        n163 = Scan From String(format string="%f", input string=w973) -> (output 1=w976:dbl)  [unwired: 3 in, 3 out]
                        n164 = Build Array (concatenate)(w974, w976) -> (w975:dbl[])
                      }
                    }
                    frame #4 {
                      n165 = VISA Write(VISA resource name=w984, write buffer=":ABORT;\n:OUTP OFF;\n*RST" ("data"), error in (no error)=w983) -> (VISA resource name out=w978:refnum<visa-resource-name>, error out=w981:errorcluster)  [unwired: 1 out]
                    }
                    frame #5 {
                      n166 = VISA Write(VISA resource name=w988, write buffer=":STAT:PRES;\n:*CLS" ("data"), error in (no error)=w987) -> (VISA resource name out=w985:refnum<visa-resource-name>, error out=w986:errorcluster)  [unwired: 1 out]
                    }
                  }
                  n167 = call-poly <vilib>:"Mean.vi"("X"=w848) -> ("mean"=w872:dbl, "error"=w860:i32)
                  n168 = Number To Engineering String(4:w860) -> (0:w859:string)  [unwired: 3 in]
                  n169 = call-poly <vilib>:"Mean.vi"("X"=w847) -> ("mean"=w871:dbl, "error"=w864:i32)
                  n170 = Divide(x=w872, y=w871) -> (x/y=w870:dbl)
                  n171 = Number To Engineering String(4:w864) -> (0:w863:string)  [unwired: 3 in]
                  n172 = Build Array(w872, w871, w870) -> (w873:dbl[])
                  n173 = Number To Engineering String(4:w871) -> (0:w865:string)  [unwired: 3 in]
                  n174 = Number To Engineering String(4:w870) -> (0:w857:string)  [unwired: 3 in]
                  n175 = Number To Engineering String(4:w872) -> (0:w861:string)  [unwired: 3 in]
                  n176 = Concatenate Strings("Measured Source current: " ("string"), w865, w863, " measured voltage: " ("string"), w861, w859, " calculated resistance: " ("string"), w857) -> (w869:string)
                }
                frame "SR830" {
                }
                frame "SR830 and 6221" {
                }
              }
              n177 = Concatenate Strings(w768, w774, w770) -> (w772:string)
              "Measurement Log" <- w772
              n178 = call "add measurements to map.vi"("Measurement Values"=w766, "Measurement Names"=w767, "Measurements Map in"=w765) -> ("Measurements Map Out"=w763:map{string, dbl[]})  [unwired: 2 in]
              n179 = for {
                tunnel: [w793] -> _ mode=indexing
                tunnel: w763 -> [w793] mode=indexing
                tunnel: [w792] -> w762 mode=indexing
                tunnel: [w791] -> w761 mode=indexing
                n180 = Unbundle(w793) -> (w792:string, "Array"=w791:dbl[])
              }
              "Results Description" <- w762
              n181 = Search and Replace String(replace all?=TRUE, input string=w772, search string=w770) -> (number of replacements=w769:i32)  [unwired: 5 in, 3 out]
              n182 = property on="Measurement Log" class="Str"("Text.Scroll Position"=w769) -> ()  [unwired: 2 in, 2 out]
              n183 = Transpose 2D Array(2D array=w761) -> (transposed array=→"Results":dbl[][])
              n184 = Array Size(array=w762) -> (size(s)=w764:i32)
              n185 = property on="Results" class="Arr (strict)"("Number of Columns"=w764) -> ()  [unwired: 2 in, 2 out]
              n186 = property on="Results Description" class="Arr (strict)"("Number of Columns"=w764) -> ()  [unwired: 2 in, 2 out]
            }
            n187 = VISA Write(VISA resource name=w687, write buffer="ROUT:OPEN:ALL", error in (no error)=w669) -> (VISA resource name out=w686:refnum<visa-resource-name>, error out=w685:errorcluster)  [unwired: 1 out]
            n188 = case shown="\"2400 and  2182\"" w703 {
              tunnel: w702 -> [_ w722 w727 _ _]
              tunnel: w701 -> [w718 w721 w728 _ _]
              tunnel: [w718 w720 w723 _ _] -> w672
              tunnel: w675 -> [_ _ w726 _ _]
              tunnel: w674 -> [w717 w719 w725 _ _]
              tunnel: [w717 w719 w724 _ _] -> w671
              frame "DAQ6510", Default {
              }
              frame "2400 Only" {
                n189 = call <instrlib>:"Close.vi"("error in (no error)"=w721, "VISA resource name"=w722) -> ("error out"=w720:errorcluster)  [unwired: 9 in]
              }
              frame "2400 and  2182" {
                n190 = call <instrlib>:"Close.vi"("error in (no error)"=w728, "VISA resource name"=w727) -> ("error out"=w723:errorcluster)  [unwired: 9 in]
                n191 = call <instrlib>:"Close.vi"("error in (no error)"=w725, "VISA resource name"=w726) -> ("error out"=w724:errorcluster)  [unwired: 9 in]
              }
              frame "SR830" {
              }
              frame "SR830 and 6221" {
              }
            }
            n192 = call <instrlib>:"Close.vi"("error in (no error)"=w685, "VISA resource name"=w686) -> ("error out"=w668:errorcluster)  [unwired: 9 in]
            n193 = call "save measurements.vi"("Save path"=w691, "Measurements In"=w673) -> ()  [unwired: 12 in, 2 out]
            n194 = Build Array(w668, w672, w671) -> (→"Comms Errors":errorcluster[])
          }
        }
        n195 = case shown="\"2400 and  2182\"" "Radio Buttons" {
          tunnel: [w648 w650 w652 w653 w656] -> w641
          tunnel: [w648 w651 w652 w653 w655] -> w640
          tunnel: [TRUE w651 w652 TRUE w656] -> w636
          tunnel: [w648 w651 w652 w653 w656] -> w635
          tunnel: [w648 w650 w652 w653 w655] -> w628
          frame "DAQ6510", Default {
            w648 = FALSE
          }
          frame "2400 Only" {
            w651 = TRUE
            w650 = FALSE
          }
          frame "2400 and  2182" {
            w652 = TRUE
          }
          frame "SR830" {
            w653 = FALSE
          }
          frame "SR830 and 6221" {
            w655 = FALSE
            w656 = TRUE
          }
        }
        n196 = property on="Size Of Buffer Used For One Measurement" class="DigNum (strict)"("Visible"=w628) -> ()  [unwired: 2 in, 2 out]
        n197 = property on="Measurement Repeats" class="DigNum (strict)"("Visible"=w636) -> ()  [unwired: 2 in, 2 out]
        n198 = property on="Current (µA)" class="DigNum (strict)"("Visible"=w640) -> ()  [unwired: 2 in, 2 out]
        n199 = property on="Measure Instrument" class="VISAName"("Visible"=w641) -> ()  [unwired: 2 in, 2 out]
        n200 = property on="Compliance voltage (V)" class="DigNum (strict)"("Visible"=w635) -> ()  [unwired: 2 in, 2 out]
      }
      frame 3 {
        # "Magnetic Op."
      }
      frame 4 {
        # "Calculations"
        # "Save File - saves collected data into a (csv) file and asks for a file path if not already given"
        n201 = Look In Map(map=w1006, key="Resistance") -> (value=w1004:dbl[])  [unwired: 1 in, 1 out]
        n202 = Build Array("Top Film R est.", "Bottm Film R est.", "RA est.") -> (w1014:dbl[])
        n203 = case shown="True" "Fit Data" {
          tunnel: w1009 -> [_ w1034]
          tunnel: w1014 -> [_ w1032]
          tunnel: [dbl[] [0.0, 0.0, 0.0] w1023] -> w1011
          tunnel: w1004 -> [_ w1021]
          frame False {
          }
          frame True {
            # "Calculated R"
            # "Mean probe spacing"
            n204 = Index Array(array=w1034, index (col)=4 ("disabled index (col)")) -> (element=w1033:i64[])  [unwired: 1 in]
            n205 = vi-ref "modelFunction.vi"() -> (w1031:refnum<vi>)
            n206 = call-poly <vilib>:"Nonlinear Curve Fit.vi"("Y"=w1021, "f(x,a)"=w1031, "X"=w1033, "initial parameters"=w1032) -> ("best fit parameters"=w1023:dbl[], "error out"=→"error out (fitting model)":errorcluster)  [unwired: 6 in, 4 out]
            n207 = Index Array(array=w1023, index=0) -> (element=→"Top Film R":dbl)
            n208 = Index Array(array=w1023, index=1) -> (element=→"Bottom Film R":dbl)
            n209 = Index Array(array=w1023, index=2) -> (element=→"RA":dbl)
          }
        }
        n210 = case shown="True" "Save File" {
          tunnel: w1009 -> [_ w1055]
          tunnel: string[] ["I+", "V+", "V-", "I-", "x (mean probe spacing)", "V", "I (µA)", "R (=V/I)"] -> [_ w1051]
          tunnel: string[] ["R (t)", "R (b)", "RA"] -> [_ w1043]
          tunnel: w1011 -> [_ w1036]
          tunnel: w1007 -> [_ w1035]
          frame False {
          }
          frame True {
            n211 = call-poly <vilib>:"Write Delimited Spreadsheet.vi"("file path (dialog if empty)"=w1035, "1D data"=w1051, "delimiter (\\t)"="," ("delimiter (\\t)")) -> ("new file path (Not A Path if cancelled)"=w1053:path, "error out"=w1052:errorcluster)  [unwired: 11 in]
            n212 = call-poly <vilib>:"Write Delimited Spreadsheet.vi"("file path (dialog if empty)"=w1053, "format (%d)"="%.6f" ("format (%.3f)"), "2D data"=w1055, "append to file? (new file:F)"=TRUE, "error in (no error)"=w1052, "delimiter (\\t)"="," ("delimiter (\\t)")) -> ("new file path (Not A Path if cancelled)"=w1045:path, "error out"=w1044:errorcluster)  [unwired: 8 in]
            n213 = call-poly <vilib>:"Write Delimited Spreadsheet.vi"("file path (dialog if empty)"=w1045, "format (%s)"="%.6f" ("format (%.3f)"), "1D data"=w1043, "append to file? (new file:F)"=TRUE, "error in (no error)"=w1044, "delimiter (\\t)"="," ("delimiter (\\t)")) -> ("new file path (Not A Path if cancelled)"=w1038:path, "error out"=w1037:errorcluster)  [unwired: 8 in]
            n214 = call-poly <vilib>:"Write Delimited Spreadsheet.vi"("file path (dialog if empty)"=w1038, "format (%.3f)"="%.6f", "1D data"=w1036, "append to file? (new file:F)"=TRUE, "error in (no error)"=w1037, "delimiter (\\t)"="," ("delimiter (\\t)")) -> ("error out"=→"error file out":errorcluster)  [unwired: 8 in, 1 out]
          }
        }
        "Measurements Map Out" <- w1006
      }
    }
    n215 = case shown="False" "Exit Camera 2" {
      tunnel: ["" "Exit camera"] -> w241
      frame False {
      }
      frame True {
      }
    }
    n216 = case shown="False" "Init Camera 2" {
      tunnel: ["" "Init camera"] -> w244
      frame False {
      }
      frame True {
      }
    }
    n217 = case shown="False" "Init Camera" {
      tunnel: ["" "Init camera"] -> w257
      frame False {
      }
      frame True {
      }
    }
    n218 = case shown="False" "Exit Camera" {
      tunnel: ["" "Exit camera"] -> w254
      frame False {
      }
      frame True {
      }
    }
    n219 = property on="Image first camera" class="Pict"("ZoomFactor"=0.175) -> ()  [unwired: 2 in, 2 out]
    n220 = property on="Image second camera" class="Pict"("ZoomFactor"=0.175) -> ()  [unwired: 2 in, 2 out]
    n221 = Concatenate Strings(w244, w241) -> (w243:string)
    n222 = Concatenate Strings(w257, w254) -> (w256:string)
    n223 = case shown="\"Init camera\"" w243 {
      tunnel: w234 -> [w385 w416 w481]
      tunnel: w233 -> [w386 w415 w480]
      tunnel: [w395 w418 w459] -> w236
      tunnel: [w396 w417 w460] -> w240
      tunnel: [TRUE FALSE FALSE] -> w238
      frame "Exit camera" {
        # "Close .Net Referenz"
        # "Is acquisition running?"
        # "Stop Acquisition"
        # "Close Camera"
        n224 = control-ref of="Init Camera 2"() -> (w380:refnum<vi>)
        n225 = control-ref of="Exit Camera 2"() -> (w379:refnum<vi>)
        n226 = property class="Camera"(reference=w385, error in=w386) -> (error out=w394:errorcluster, "Acquisition"=w393:refnum<k24>)  [unwired: 1 out]
        n227 = property class="Bool"(reference=w380, "Disabled"=u8 0 ("Deaktiviert")) -> ()  [unwired: 1 in, 2 out]
        n228 = property class="Bool"(reference=w379, "Disabled"=u8 2 ("Deaktiviert")) -> ()  [unwired: 1 in, 2 out]
        n229 = invoke class="Acquisition" method="HasStarted"(reference=w393, error in=w394) -> (reference out=w387:refnum<k24>, error out=w390:errorcluster, "bValue"=w392:bool)  [unwired: 2 in, 1 out]
        n230 = invoke class="Acquisition" method="ToString"(reference=w387, error in=w390) -> (error out=w389:errorcluster, "ToString"=w388:string)  [unwired: 1 in, 1 out]
        n231 = call <instrlib>:"Error_Handling.vi"("Error String"=w388, "Error In"=w389) -> ("Error Out"=w391:errorcluster)  [unwired: 9 in]
        n232 = case shown="True" w392 {
          tunnel: [w404 w413] -> w383
          tunnel: w391 -> [w404 w414]
          tunnel: w385 -> [w403 w405]
          tunnel: [w403 w405] -> w384
          frame False {
          }
          frame True {
            n233 = property class="Camera"(reference=w405, error in=w414) -> (error out=w409:errorcluster, "Acquisition"=w410:refnum<k24>)  [unwired: 1 out]
            n234 = invoke class="Acquisition" method="Stop"(reference=w410, error in=w409) -> (reference out=w407:refnum<k24>, error out=w408:errorcluster, "Stop"=w406:i32)  [unwired: 1 in]
            n235 = invoke class="Acquisition" method="ToString"(reference=w407, error in=w408) -> (error out=w412:errorcluster, "ToString"=w411:string)  [unwired: 1 in, 1 out]
            n236 = call <instrlib>:"Error_Handling.vi"("Error Code"=w406, "Error String"=w411, "Error In"=w412) -> ("Error Out"=w413:errorcluster)  [unwired: 8 in]
          }
        }
        n237 = invoke class="Camera" method="Exit"(reference=w384, error in=w383) -> (reference out=w395:refnum<k24>, error out=w399:errorcluster, "Exit"=w398:i32)  [unwired: 1 in]
        n238 = invoke class="Camera" method="ToString"(reference=w395, error in=w399) -> (error out=w400:errorcluster, "ToString"=w401:string)  [unwired: 1 in, 1 out]
        n239 = call <instrlib>:"Error_Handling.vi"("Error Code"=w398, "Error String"=w401, "Error In"=w400) -> ("Error Out"=w397:errorcluster)  [unwired: 8 in]
        n240 = Close Reference ("Close Referenz")(reference=w395, error in (no error)=w397) -> (error out=w396:errorcluster)
      }
      frame Default {
        # "Has acquisition started?"
        # "Show Image"
        n241 = property class="Camera"(reference=w416, error in=w415) -> (error out=w427:errorcluster, "Acquisition"=w426:refnum<k24>)  [unwired: 1 out]
        n242 = invoke class="Acquisition" method="HasStarted"(reference=w426, error in=w427) -> (reference out=w422:refnum<k24>, error out=w421:errorcluster, "HasStarted"=w420:i32, "bValue"=w425:bool)  [unwired: 2 in]
        n243 = invoke class="Acquisition" method="ToString"(reference=w422, error in=w421) -> (error out=w424:errorcluster, "ToString"=w423:string)  [unwired: 1 in, 1 out]
        n244 = call <instrlib>:"Error_Handling.vi"("Error Code"=w420, "Error String"=w423, "Error In"=w424) -> ("Error Out"=w419:errorcluster)  [unwired: 8 in]
        n245 = case shown="False" w425 {
          tunnel: [w430 w436] -> w417
          tunnel: w419 -> [w430 w435]
          tunnel: w416 -> [w429 w431]
          tunnel: [w429 w431] -> w418
          frame False {
          }
          frame True {
            # "Memory"
            n246 = property class="Camera"(reference=w431, error in=w435) -> (error out=w438:errorcluster, "Memory"=w439:refnum<k24>)  [unwired: 1 out]
            n247 = invoke class="Memory" method="GetActive"(reference=w439, error in=w438) -> (reference out=w445:refnum<k24>, error out=w444:errorcluster, "GetActive"=w446:i32, "s32MemId"=w437:i32)  [unwired: 2 in]
            n248 = invoke class="Memory" method="ToString"(reference=w445, error in=w444) -> (error out=w442:errorcluster, "ToString"=w443:string)  [unwired: 1 in, 1 out]
            n249 = call <instrlib>:"Error_Handling.vi"("Error Code"=w446, "Error String"=w443, "Error In"=w442) -> ("Error Out"=w447:errorcluster)  [unwired: 8 in]
            n250 = property class="Camera"(reference=w431, error in=w447) -> (error out=w441:errorcluster, "Memory"=w440:refnum<k24>)  [unwired: 1 out]
            n251 = invoke class="Memory" method="CopyToArray"(reference=w440, error in=w441, "s32MemId"=w437) -> (reference out=w450:refnum<k24>, error out=w451:errorcluster, "CopyToArray"=w452:i32, "u8Image"=w432:u8[])  [unwired: 2 in, 1 out]
            n252 = invoke class="Memory" method="ToString"(reference=w450, error in=w451) -> (error out=w448:errorcluster, "ToString"=w449:string)  [unwired: 1 in, 1 out]
            n253 = call <instrlib>:"Error_Handling.vi"("Error Code"=w452, "Error String"=w449, "Error In"=w448) -> ("Error Out"=w433:errorcluster)  [unwired: 8 in]
            n254 = call <instrlib>:"ArrayToImage.vi"("Error In"=w433, "InArray"=w432, ".NET (Reference)"=w431) -> ("Error Out"=w436:errorcluster, "Image"=→"Image second camera":picture)  [unwired: 7 in]
          }
        }
      }
      frame "Init camera" {
        w461 = 1 items=["IS_DONT_WAIT", "IS_WAIT"] ("Wait")
        w488 = 0 items=["RGB 32"=0, "RGB 24"=1, "Y8 Monochrom"=6] ("Mode")
        # "SubVI Example for \nGetDefault Timing"
        # "SubVI Example for \nMemory allocation"
        # "SubVI Example for \nTiming"
        # "SubVI Example for \nCamera Init"
        # "Pixelformat"
        n255 = control-ref of="Init Camera 2"() -> (w456:refnum<vi>)
        n256 = control-ref of="Exit Camera 2"() -> (w454:refnum<vi>)
        n257 = property class="Bool"(reference=w456, "Disabled"=u8 2 ("Deaktiviert")) -> ()  [unwired: 1 in, 2 out]
        n258 = property class="Bool"(reference=w454, "Disabled"=u8 0 ("Deaktiviert")) -> ()  [unwired: 1 in, 2 out]
        n259 = call <instrlib>:"SubVI_Example_CameraInit.vi"("Error In"=w480, "Camera ID"="Camera ID 3", "Init Camera Flag"=TRUE, ".NET (Reference)"=w481) -> ("Error Out"=w485:errorcluster, ".NET (Reference)"=w459:refnum<k24>)  [unwired: 6 in]
        n260 = property class="Camera"(reference=w459, error in=w485) -> (error out=w486:errorcluster, "PixelFormat"=w487:refnum<k24>)  [unwired: 1 out]
        n261 = invoke class="PixelFormat" method="Set"(reference=w487, error in=w486, "mode"=w488) -> (reference out=w483:refnum<k24>, error out=w477:errorcluster, "Set"=w482:i32)  [unwired: 1 in, 1 out]
        n262 = invoke class="PixelFormat" method="ToString"(reference=w483, error in=w477) -> (error out=w476:errorcluster, "ToString"=w484:string)  [unwired: 1 in, 1 out]
        n263 = call <instrlib>:"Error_Handling.vi"("Error Code"=w482, "Error String"=w484, "Error In"=w476) -> ("Error Out"=w473:errorcluster)  [unwired: 8 in]
        n264 = call <instrlib>:"SubVI_Example_GetDefault_Timing.vi"(".NET (Reference)"=w459, "Error In"=w473) -> ("Pixelclock"=w470:i32, "Exposure time"=w471:dbl, "Framerate"=w472:dbl, "Error Out"=w469:errorcluster)  [unwired: 10 in]
        n265 = call <instrlib>:"SubVI_Example_Timing.vi"(".NET (Reference)"=w459, "Pixelclock"=w470, "Exposure time"=w471, "Framerate"=w472, "Error In"=w469) -> ("Error Out"=w475:errorcluster)  [unwired: 7 in, 3 out]
        n266 = call <instrlib>:"SubVI_Example_MemoryAllocation.vi"(".NET (Reference)"=w459, "Error In"=w475) -> ("Serial Number"=→"Serial Number 2":string, "Error Out"=w458:errorcluster)  [unwired: 13 in, 3 out]
        n267 = property class="Camera"(reference=w459, error in=w458) -> (error out=w467:errorcluster, "Acquisition"=w468:refnum<k24>)  [unwired: 1 out]
        n268 = invoke class="Acquisition" method="Capture"(reference=w468, error in=w467, "param"=w461) -> (reference out=w463:refnum<k24>, error out=w464:errorcluster, "Capture"=w462:i32)  [unwired: 1 in, 1 out]
        n269 = invoke class="Acquisition" method="ToString"(reference=w463, error in=w464) -> (error out=w466:errorcluster, "ToString"=w465:string)  [unwired: 1 in, 1 out]
        n270 = call <instrlib>:"Error_Handling.vi"("Error Code"=w462, "Error String"=w465, "Error In"=w466) -> ("Error Out"=w460:errorcluster)  [unwired: 8 in]
      }
    }
    n271 = case shown="Default" w256 {
      tunnel: w247 -> [w499 w530 w595]
      tunnel: w246 -> [w500 w529 w594]
      tunnel: [w509 w532 w574] -> w249
      tunnel: [w510 w531 w575] -> w253
      tunnel: [TRUE FALSE FALSE] -> w251
      frame "Exit camera" {
        # "Close .Net Referenz"
        # "Is acquisition running?"
        # "Stop Acquisition"
        # "Close Camera"
        n272 = control-ref of="Init Camera"() -> (w494:refnum<vi>)
        n273 = control-ref of="Exit Camera"() -> (w493:refnum<vi>)
        n274 = property class="Camera"(reference=w499, error in=w500) -> (error out=w508:errorcluster, "Acquisition"=w507:refnum<k24>)  [unwired: 1 out]
        n275 = property class="Bool"(reference=w494, "Disabled"=u8 0 ("Deaktiviert")) -> ()  [unwired: 1 in, 2 out]
        n276 = property class="Bool"(reference=w493, "Disabled"=u8 2 ("Deaktiviert")) -> ()  [unwired: 1 in, 2 out]
        n277 = invoke class="Acquisition" method="HasStarted"(reference=w507, error in=w508) -> (reference out=w501:refnum<k24>, error out=w504:errorcluster, "bValue"=w506:bool)  [unwired: 2 in, 1 out]
        n278 = invoke class="Acquisition" method="ToString"(reference=w501, error in=w504) -> (error out=w503:errorcluster, "ToString"=w502:string)  [unwired: 1 in, 1 out]
        n279 = call <instrlib>:"Error_Handling.vi"("Error String"=w502, "Error In"=w503) -> ("Error Out"=w505:errorcluster)  [unwired: 9 in]
        n280 = case shown="True" w506 {
          tunnel: [w518 w527] -> w497
          tunnel: w505 -> [w518 w528]
          tunnel: w499 -> [w517 w519]
          tunnel: [w517 w519] -> w498
          frame False {
          }
          frame True {
            n281 = property class="Camera"(reference=w519, error in=w528) -> (error out=w523:errorcluster, "Acquisition"=w524:refnum<k24>)  [unwired: 1 out]
            n282 = invoke class="Acquisition" method="Stop"(reference=w524, error in=w523) -> (reference out=w521:refnum<k24>, error out=w522:errorcluster, "Stop"=w520:i32)  [unwired: 1 in]
            n283 = invoke class="Acquisition" method="ToString"(reference=w521, error in=w522) -> (error out=w526:errorcluster, "ToString"=w525:string)  [unwired: 1 in, 1 out]
            n284 = call <instrlib>:"Error_Handling.vi"("Error Code"=w520, "Error String"=w525, "Error In"=w526) -> ("Error Out"=w527:errorcluster)  [unwired: 8 in]
          }
        }
        n285 = invoke class="Camera" method="Exit"(reference=w498, error in=w497) -> (reference out=w509:refnum<k24>, error out=w513:errorcluster, "Exit"=w512:i32)  [unwired: 1 in]
        n286 = invoke class="Camera" method="ToString"(reference=w509, error in=w513) -> (error out=w514:errorcluster, "ToString"=w515:string)  [unwired: 1 in, 1 out]
        n287 = call <instrlib>:"Error_Handling.vi"("Error Code"=w512, "Error String"=w515, "Error In"=w514) -> ("Error Out"=w511:errorcluster)  [unwired: 8 in]
        n288 = Close Reference ("Close Referenz")(reference=w509, error in (no error)=w511) -> (error out=w510:errorcluster)
      }
      frame Default {
        # "Has acquisition started?"
        n289 = property class="Camera"(reference=w530, error in=w529) -> (error out=w541:errorcluster, "Acquisition"=w540:refnum<k24>)  [unwired: 1 out]
        n290 = invoke class="Acquisition" method="HasStarted"(reference=w540, error in=w541) -> (reference out=w536:refnum<k24>, error out=w535:errorcluster, "HasStarted"=w534:i32, "bValue"=w539:bool)  [unwired: 2 in]
        n291 = invoke class="Acquisition" method="ToString"(reference=w536, error in=w535) -> (error out=w538:errorcluster, "ToString"=w537:string)  [unwired: 1 in, 1 out]
        n292 = call <instrlib>:"Error_Handling.vi"("Error Code"=w534, "Error String"=w537, "Error In"=w538) -> ("Error Out"=w533:errorcluster)  [unwired: 8 in]
        n293 = case shown="True" w539 {
          tunnel: [w544 w550] -> w531
          tunnel: w533 -> [w544 w549]
          tunnel: w530 -> [w543 w547]
          tunnel: [w543 w547] -> w532
          frame False {
            # "Show Image"
          }
          frame True {
            # "Memory"
            n294 = property class="Camera"(reference=w547, error in=w549) -> (error out=w552:errorcluster, "Memory"=w553:refnum<k24>)  [unwired: 1 out]
            n295 = invoke class="Memory" method="GetActive"(reference=w553, error in=w552) -> (reference out=w559:refnum<k24>, error out=w558:errorcluster, "GetActive"=w560:i32, "s32MemId"=w551:i32)  [unwired: 2 in]
            n296 = invoke class="Memory" method="ToString"(reference=w559, error in=w558) -> (error out=w556:errorcluster, "ToString"=w557:string)  [unwired: 1 in, 1 out]
            n297 = call <instrlib>:"Error_Handling.vi"("Error Code"=w560, "Error String"=w557, "Error In"=w556) -> ("Error Out"=w561:errorcluster)  [unwired: 8 in]
            n298 = property class="Camera"(reference=w547, error in=w561) -> (error out=w555:errorcluster, "Memory"=w554:refnum<k24>)  [unwired: 1 out]
            n299 = invoke class="Memory" method="CopyToArray"(reference=w554, error in=w555, "s32MemId"=w551) -> (reference out=w564:refnum<k24>, error out=w565:errorcluster, "CopyToArray"=w566:i32, "u8Image"=w546:u8[])  [unwired: 2 in, 1 out]
            n300 = invoke class="Memory" method="ToString"(reference=w564, error in=w565) -> (error out=w562:errorcluster, "ToString"=w563:string)  [unwired: 1 in, 1 out]
            n301 = call <instrlib>:"Error_Handling.vi"("Error Code"=w566, "Error String"=w563, "Error In"=w562) -> ("Error Out"=w548:errorcluster)  [unwired: 8 in]
            n302 = call <instrlib>:"ArrayToImage.vi"("Error In"=w548, "InArray"=w546, ".NET (Reference)"=w547) -> ("Error Out"=w550:errorcluster, "Image"=→"Image first camera":picture)  [unwired: 7 in]
          }
        }
      }
      frame "Init camera" {
        w576 = 1 items=["IS_DONT_WAIT", "IS_WAIT"] ("Wait")
        w602 = 0 items=["RGB 32"=0, "RGB 24"=1, "Y8 Monochrom"=6] ("Mode")
        # "SubVI Example for \nGetDefault Timing"
        # "SubVI Example for \nMemory allocation"
        # "SubVI Example for \nTiming"
        # "SubVI Example for \nCamera Init"
        # "Pixelformat"
        n303 = control-ref of="Init Camera"() -> (w570:refnum<vi>)
        n304 = control-ref of="Exit Camera"() -> (w568:refnum<vi>)
        n305 = call <instrlib>:"SubVI_Example_CameraInit.vi"("Error In"=w594, "Camera ID"="Camera ID 1", "Init Camera Flag"=TRUE, ".NET (Reference)"=w595) -> ("Error Out"=w599:errorcluster, ".NET (Reference)"=w574:refnum<k24>)  [unwired: 6 in]
        n306 = property class="Bool"(reference=w570, "Disabled"=u8 2 ("Deaktiviert")) -> ()  [unwired: 1 in, 2 out]
        n307 = property class="Bool"(reference=w568, "Disabled"=u8 0 ("Deaktiviert")) -> ()  [unwired: 1 in, 2 out]
        n308 = property class="Camera"(reference=w574, error in=w599) -> (error out=w600:errorcluster, "PixelFormat"=w601:refnum<k24>)  [unwired: 1 out]
        n309 = invoke class="PixelFormat" method="Set"(reference=w601, error in=w600, "mode"=w602) -> (reference out=w597:refnum<k24>, error out=w591:errorcluster, "Set"=w596:i32)  [unwired: 1 in, 1 out]
        n310 = invoke class="PixelFormat" method="ToString"(reference=w597, error in=w591) -> (error out=w590:errorcluster, "ToString"=w598:string)  [unwired: 1 in, 1 out]
        n311 = call <instrlib>:"Error_Handling.vi"("Error Code"=w596, "Error String"=w598, "Error In"=w590) -> ("Error Out"=w587:errorcluster)  [unwired: 8 in]
        n312 = call <instrlib>:"SubVI_Example_GetDefault_Timing.vi"(".NET (Reference)"=w574, "Error In"=w587) -> ("Pixelclock"=w584:i32, "Exposure time"=w585:dbl, "Framerate"=w586:dbl, "Error Out"=w572:errorcluster)  [unwired: 10 in]
        n313 = call <instrlib>:"SubVI_Example_Timing.vi"(".NET (Reference)"=w574, "Pixelclock"=w584, "Exposure time"=w585, "Framerate"=w586, "Error In"=w572) -> ("Error Out"=w589:errorcluster)  [unwired: 7 in, 3 out]
        n314 = call <instrlib>:"SubVI_Example_MemoryAllocation.vi"(".NET (Reference)"=w574, "Error In"=w589) -> ("Serial Number"=→"Serial Number 1":string, "Error Out"=w573:errorcluster)  [unwired: 13 in, 3 out]
        n315 = property class="Camera"(reference=w574, error in=w573) -> (error out=w582:errorcluster, "Acquisition"=w583:refnum<k24>)  [unwired: 1 out]
        n316 = invoke class="Acquisition" method="Capture"(reference=w583, error in=w582, "param"=w576) -> (reference out=w578:refnum<k24>, error out=w579:errorcluster, "Capture"=w577:i32)  [unwired: 1 in, 1 out]
        n317 = invoke class="Acquisition" method="ToString"(reference=w578, error in=w579) -> (error out=w581:errorcluster, "ToString"=w580:string)  [unwired: 1 in, 1 out]
        n318 = call <instrlib>:"Error_Handling.vi"("Error Code"=w577, "Error String"=w580, "Error In"=w581) -> ("Error Out"=w575:errorcluster)  [unwired: 8 in]
      }
    }
    n319 = case shown="False" "steps /\n continuous \ntoggle" {
      tunnel: w220 -> [w277 w353]
      tunnel: w219 -> [w276 w352]
      tunnel: [w295 w359] -> w218
      tunnel: [w268 w365] -> w208
      tunnel: "up a1" -> [w294 w361]
      tunnel: "down a1" -> [w292 w360]
      tunnel: "up all" -> [w275 w348]
      tunnel: "down all" -> [w274 w349]
      tunnel: "down a3" -> [w282 w357]
      tunnel: "up a3" -> [w283 w356]
      tunnel: "down a2" -> [w280 w351]
      tunnel: "up a2" -> [w281 w350]
      tunnel: w213 -> [_ w363]
      tunnel: [_ w364] -> w217
      tunnel: [_ w344] -> w216
      tunnel: w212 -> [_ w341]
      tunnel: [_ w342] -> w214
      tunnel: w210 -> [_ w339]
      tunnel: [_ w343] -> w215
      tunnel: w211 -> [_ w340]
      frame False {
        n320 = flat-sequence {
          tunnel: w277 -> [w310]
          tunnel: w276 -> [w313]
          tunnel: w283 -> [w308]
          tunnel: "a3" ("Combo Box") -> [w306]
          tunnel: "Step size" -> [w309]
          tunnel: w282 -> [w307]
          tunnel: [w312] -> w286
          tunnel: [w311] -> w285
          tunnel: [w315] -> _
          tunnel: [w316] -> w270
          tunnel: w286 -> [w316]
          tunnel: w285 -> [w315]
          frame #0 {
            n321 = call "Picomotor step single.vi"("Step size"=w309, "Combo Box"=w306, "error in (no error)"=w313, "down a1"=w307, "up a1"=w308, "VISA Refnum in"=w310) -> ("error out"=w312:errorcluster, "VISA Refnum out"=w311:refnum<visa-resource-name>)  [unwired: 4 in]
          }
          frame #1 {
            n322 = Wait (ms)(milliseconds to wait=u32 100) -> ()  [unwired: 1 out]
          }
        }
        n323 = flat-sequence {
          tunnel: w277 -> [w332]
          tunnel: w276 -> [w335]
          tunnel: w294 -> [w330]
          tunnel: "a1" ("Combo Box") -> [w328]
          tunnel: "Step size" -> [w331]
          tunnel: w292 -> [w329]
          tunnel: [w334] -> w291
          tunnel: [w333] -> w290
          tunnel: [w337] -> w295
          tunnel: [w338] -> w272
          tunnel: w291 -> [w338]
          tunnel: w290 -> [w337]
          frame #0 {
            n324 = call "Picomotor step single.vi"("Step size"=w331, "Combo Box"=w328, "error in (no error)"=w335, "down a1"=w329, "up a1"=w330, "VISA Refnum in"=w332) -> ("error out"=w334:errorcluster, "VISA Refnum out"=w333:refnum<visa-resource-name>)  [unwired: 4 in]
          }
          frame #1 {
            n325 = Wait (ms)(milliseconds to wait=u32 100) -> ()  [unwired: 1 out]
          }
        }
        n326 = flat-sequence {
          tunnel: w277 -> [w321]
          tunnel: w276 -> [w324]
          tunnel: w281 -> [w319]
          tunnel: "a2" ("Combo Box") -> [w317]
          tunnel: "Step size" -> [w320]
          tunnel: w280 -> [w318]
          tunnel: [w323] -> w289
          tunnel: [w322] -> w288
          tunnel: [w326] -> _
          tunnel: [w327] -> w271
          tunnel: w289 -> [w327]
          tunnel: w288 -> [w326]
          frame #0 {
            n327 = call "Picomotor step single.vi"("Step size"=w320, "Combo Box"=w317, "error in (no error)"=w324, "down a1"=w318, "up a1"=w319, "VISA Refnum in"=w321) -> ("error out"=w323:errorcluster, "VISA Refnum out"=w322:refnum<visa-resource-name>)  [unwired: 4 in]
          }
          frame #1 {
            n328 = Wait (ms)(milliseconds to wait=u32 100) -> ()  [unwired: 1 out]
          }
        }
        n329 = flat-sequence {
          tunnel: [w302] -> w279
          tunnel: [w301] -> w278
          tunnel: w277 -> [w300]
          tunnel: w276 -> [w299]
          tunnel: w275 -> [w298]
          tunnel: w274 -> [w297]
          tunnel: "Step size" -> [w296]
          tunnel: [w304] -> _
          tunnel: [w305] -> w269
          tunnel: w279 -> [w305]
          tunnel: w278 -> [w304]
          frame #0 {
            n330 = call "Picomotor step multi.vi"("Step size"=w296, "error in (no error)"=w299, "down a1"=w297, "up a1"=w298, "VISA Refnum in"=w300) -> ("error out"=w302:errorcluster, "VISA Refnum out"=w301:refnum<visa-resource-name>)  [unwired: 5 in]
          }
          frame #1 {
            n331 = Wait (ms)(milliseconds to wait=u32 100) -> ()  [unwired: 1 out]
          }
        }
        n332 = Merge Errors(w272, w271, w270, w269) -> (w268:errorcluster)
      }
      frame True {
        n333 = call "Picomotor single motor continuous.vi"("Enum"=w363, "Combo Box"="a1", "error in (no error)"=w352, "down"=w360, "up"=w361, "VISA Refnum in"=w353) -> ("error out"=w358:errorcluster, "Numeric"=w364:i32, "VISA Refnum out"=w359:refnum<visa-resource-name>)  [unwired: 3 in]
        n334 = call "Picomotor single motor continuous.vi"("Enum"=w340, "Combo Box"="a3", "error in (no error)"=w352, "down"=w357, "up"=w356, "VISA Refnum in"=w353) -> ("error out"=w346:errorcluster, "Numeric"=w343:i32)  [unwired: 3 in, 1 out]
        n335 = call "Picomotor single motor continuous.vi"("Enum"=w341, "Combo Box"="a2", "error in (no error)"=w352, "down"=w351, "up"=w350, "VISA Refnum in"=w353) -> ("error out"=w347:errorcluster, "Numeric"=w344:i32)  [unwired: 3 in, 1 out]
        n336 = call "Picomotor all motors continuous.vi"("Enum"=w339, "error in (no error)"=w352, "down"=w349, "up"=w348, "VISA Refnum in"=w353) -> ("error out"=w345:errorcluster, "Numeric"=w342:i32)  [unwired: 4 in, 1 out]
        n337 = Merge Errors(w358, w347, w346, w345) -> (w365:errorcluster)
      }
    }
    n338 = call <instrlib>:"SubVI_Example_SyncEventLoop.vi"("Error In"=w240, "use sync"=w238, ".NET (Reference)"=w236) -> ("Error Out"=w235:errorcluster, "Synchronize (ms)"=w239:dbl)  [unwired: 7 in]
    "Error Camera 2" <- w235
    n339 = call <instrlib>:"SubVI_Example_SyncEventLoop.vi"("Error In"=w253, "use sync"=w251, ".NET (Reference)"=w249) -> ("Error Out"=w248:errorcluster, "Synchronize (ms)"=w252:dbl)  [unwired: 7 in]
    "Error Camera 1" <- w248
    n340 = Wait Until Next ms Multiple(millisecond multiple=w252) -> ()  [unwired: 1 out]
    n341 = Wait Until Next ms Multiple(millisecond multiple=w239) -> ()  [unwired: 1 out]
    n342 = case shown="True" "stop" {
      tunnel: w218 -> [w368 w373]
      tunnel: w208 -> [w367 w372]
      tunnel: [w368 w371] -> w207
      tunnel: [w367 w370] -> w209
      tunnel: [w366 w369] -> w231
      tunnel: "stop" -> [w366 w369]
      frame False {
      }
      frame True {
        n343 = call "Picomotor Write.vi"("error in (no error)"=w372, "String 3"="sto", "VISA Refnum in"=w373) -> ("error out"=w370:errorcluster, "VISA Refnum out"=w371:refnum<visa-resource-name>)  [unwired: 6 in, 1 out]
      }
    }
    n344 = Merge Errors(w209, w208) -> (w232:errorcluster)
  }
  n345 = VISA Close(VISA resource name=w1, error in (no error)=w2) -> (error out=→"error":errorcluster)
